vi "print HP.vi"(0 "peaks graph 1":cluster{cluster{"X":dbl, "Y":dbl}[]}[](graph)=[{[{"X"=0.0, "Y"=88.0}, {"X"=0.05, "Y"=88.0}, {"X"=0.1, "Y"=87.0}, {"X"=0.15000000000000002, "Y"=87.0}, {"X"=0.2, "Y"=88.0}, {"X"=0.25, "Y"=88.0}, {"X"=0.30000000000000004, "Y"=88.0}, {"X"=0.35000000000000003, "Y"=87.0}, {"X"=0.4, "Y"=88.0}, {"X"=0.45, "Y"=87.0}, {"X"=0.5, "Y"=88.0}, {"X"=0.55, "Y"=88.0}, {"X"=0.6000000000000001, "Y"=88.0}, {"X"=0.65, "Y"=88.0}, {"X"=0.7000000000000001, "Y"=87.0}, {"X"=0.75, "Y"=88.0}, {"X"=0.8, "Y"=88.0}, {"X"=0.8500000000000001, "Y"=88.0}, {"X"=0.9, "Y"=87.0}, {"X"=0.9500000000000001, "Y"=88.0}, {"X"=1.0, "Y"=88.0}, {"X"=1.05, "Y"=88.0}, {"X"=1.1, "Y"=87.0}, {"X"=1.1500000000000001, "Y"=87.0}, {"X"=1.2000000000000002, "Y"=87.0}, {"X"=1.25, "Y"=88.0}, {"X"=1.3, "Y"=88.0}, {"X"=1.35, "Y"=87.0}, {"X"=1.4000000000000001, "Y"=87.0}, {"X"=1.4500000000000002, "Y"=88.0}, {"X"=1.5, "Y"=87.0}, {"X"=1.55, "Y"=88.0}, {"X"=1.6, "Y"=88.0}, {"X"=1.6500000000000001, "Y"=87.0}, {"X"=1.7000000000000002, "Y"=87.0}, {"X"=1.75, "Y"=87.0}, {"X"=1.8, "Y"=88.0}, {"X"=1.85, "Y"=88.0}, {"X"=1.9000000000000001, "Y"=88.0}, {"X"=1.9500000000000002, "Y"=87.0}, {"X"=2.0, "Y"=88.0}, {"X"=2.0500000000000003, "Y"=87.0}, {"X"=2.1, "Y"=87.0}, {"X"=2.15, "Y"=88.0}, {"X"=2.2, "Y"=88.0}, {"X"=2.25, "Y"=87.0}, {"X"=2.3000000000000003, "Y"=88.0}, {"X"=2.35, "Y"=88.0}, {"X"=2.4000000000000004, "Y"=88.0}, {"X"=2.45, "Y"=87.0}, {"X"=2.5, "Y"=88.0}, {"X"=2.5500000000000003, "Y"=88.0}, {"X"=2.6, "Y"=87.0}, {"X"=2.6500000000000004, "Y"=87.0}, {"X"=2.7, "Y"=87.0}, {"X"=2.75, "Y"=87.0}, {"X"=2.8000000000000003, "Y"=87.0}, {"X"=2.85, "Y"=87.0}, {"X"=2.9000000000000004, "Y"=87.0}, {"X"=2.95, "Y"=87.0}, {"X"=3.0, "Y"=87.0}, {"X"=3.0500000000000003, "Y"=87.0}, {"X"=3.1, "Y"=87.0}, {"X"=3.1500000000000004, "Y"=88.0}, {"X"=3.2, "Y"=87.0}, {"X"=3.25, "Y"=88.0}, {"X"=3.3000000000000003, "Y"=87.0}, {"X"=3.35, "Y"=87.0}, {"X"=3.4000000000000004, "Y"=87.0}, {"X"=3.45, "Y"=87.0}, {"X"=3.5, "Y"=88.0}, {"X"=3.5500000000000003, "Y"=87.0}, {"X"=3.6, "Y"=87.0}, {"X"=3.6500000000000004, "Y"=87.0}, {"X"=3.7, "Y"=88.0}, {"X"=3.75, "Y"=87.0}, {"X"=3.8000000000000003, "Y"=88.0}, {"X"=3.85, "Y"=87.0}, {"X"=3.9000000000000004, "Y"=87.0}, {"X"=3.95, "Y"=88.0}, {"X"=4.0, "Y"=88.0}, {"X"=4.05, "Y"=88.0}, {"X"=4.1000000000000005, "Y"=88.0}, {"X"=4.15, "Y"=88.0}, {"X"=4.2, "Y"=88.0}, {"X"=4.25, "Y"=87.0}, {"X"=4.3, "Y"=87.0}, {"X"=4.3500000000000005, "Y"=88.0}, {"X"=4.4, "Y"=87.0}, {"X"=4.45, "Y"=87.0}, {"X"=4.5, "Y"=88.0}, {"X"=4.55, "Y"=87.0}, {"X"=4.6000000000000005, "Y"=87.0}, {"X"=4.65, "Y"=87.0}, {"X"=4.7, "Y"=87.0}, {"X"=4.75, "Y"=88.0}, {"X"=4.800000000000001, "Y"=88.0}, {"X"=4.8500000000000005, "Y"=88.0}, {"X"=4.9, "Y"=87.0}, {"X"=4.95, "Y"=87.0}, {"X"=5.0, "Y"=88.0}, {"X"=5.050000000000001, "Y"=88.0}, {"X"=5.1000000000000005, "Y"=88.0}, {"X"=5.15, "Y"=87.0}, {"X"=5.2, "Y"=88.0}, {"X"=5.25, "Y"=88.0}, {"X"=5.300000000000001, "Y"=88.0}, {"X"=5.3500000000000005, "Y"=87.0}, {"X"=5.4, "Y"=87.0}, {"X"=5.45, "Y"=87.0}, {"X"=5.5, "Y"=88.0}, {"X"=5.550000000000001, "Y"=87.0}, {"X"=5.6000000000000005, "Y"=88.0}, {"X"=5.65, "Y"=88.0}, {"X"=5.7, "Y"=88.0}, {"X"=5.75, "Y"=87.0}, {"X"=5.800000000000001, "Y"=89.0}, {"X"=5.8500000000000005, "Y"=87.0}, {"X"=5.9, "Y"=88.0}, {"X"=5.95, "Y"=88.0}, {"X"=6.0, "Y"=88.0}, {"X"=6.050000000000001, "Y"=88.0}, {"X"=6.1000000000000005, "Y"=88.0}, {"X"=6.15, "Y"=87.0}, {"X"=6.2, "Y"=88.0}, {"X"=6.25, "Y"=88.0}, {"X"=6.300000000000001, "Y"=87.0}, {"X"=6.3500000000000005, "Y"=87.0}, {"X"=6.4, "Y"=88.0}, {"X"=6.45, "Y"=87.0}, {"X"=6.5, "Y"=88.0}, {"X"=6.550000000000001, "Y"=87.0}, {"X"=6.6000000000000005, "Y"=87.0}, {"X"=6.65, "Y"=88.0}, {"X"=6.7, "Y"=87.0}, {"X"=6.75, "Y"=88.0}, {"X"=6.800000000000001, "Y"=88.0}, {"X"=6.8500000000000005, "Y"=88.0}, {"X"=6.9, "Y"=87.0}, {"X"=6.95, "Y"=87.0}, {"X"=7.0, "Y"=87.0}, {"X"=7.050000000000001, "Y"=87.0}, {"X"=7.1000000000000005, "Y"=87.0}, {"X"=7.15, "Y"=87.0}, {"X"=7.2, "Y"=87.0}, {"X"=7.25, "Y"=88.0}, {"X"=7.300000000000001, "Y"=87.0}, {"X"=7.3500000000000005, "Y"=87.0}, {"X"=7.4, "Y"=88.0}, {"X"=7.45, "Y"=87.0}, {"X"=7.5, "Y"=88.0}, {"X"=7.550000000000001, "Y"=88.0}, {"X"=7.6000000000000005, "Y"=87.0}, {"X"=7.65, "Y"=87.0}, {"X"=7.7, "Y"=87.0}, {"X"=7.75, "Y"=87.0}, {"X"=7.800000000000001, "Y"=87.0}, {"X"=7.8500000000000005, "Y"=87.0}, {"X"=7.9, "Y"=87.0}, {"X"=7.95, "Y"=88.0}, {"X"=8.0, "Y"=88.0}, {"X"=8.05, "Y"=87.0}, {"X"=8.1, "Y"=88.0}, {"X"=8.15, "Y"=87.0}, {"X"=8.200000000000001, "Y"=87.0}, {"X"=8.25, "Y"=87.0}, {"X"=8.3, "Y"=87.0}, {"X"=8.35, "Y"=86.0}, {"X"=8.4, "Y"=87.0}, {"X"=8.450000000000001, "Y"=87.0}, {"X"=8.5, "Y"=87.0}, {"X"=8.55, "Y"=87.0}, {"X"=8.6, "Y"=86.0}, {"X"=8.65, "Y"=87.0}, {"X"=8.700000000000001, "Y"=86.0}, {"X"=8.75, "Y"=87.0}, {"X"=8.8, "Y"=87.0}, {"X"=8.85, "Y"=87.0}, {"X"=8.9, "Y"=86.0}, {"X"=8.950000000000001, "Y"=86.0}, {"X"=9.0, "Y"=87.0}, {"X"=9.05, "Y"=87.0}, {"X"=9.1, "Y"=88.0}, {"X"=9.15, "Y"=87.0}, {"X"=9.200000000000001, "Y"=87.0}, {"X"=9.25, "Y"=87.0}, {"X"=9.3, "Y"=87.0}, {"X"=9.35, "Y"=87.0}, {"X"=9.4, "Y"=88.0}, {"X"=9.450000000000001, "Y"=87.0}, {"X"=9.5, "Y"=88.0}, {"X"=9.55, "Y"=87.0}, {"X"=9.600000000000001, "Y"=87.0}, {"X"=9.65, "Y"=87.0}, {"X"=9.700000000000001, "Y"=87.0}, {"X"=9.75, "Y"=87.0}, {"X"=9.8, "Y"=87.0}, {"X"=9.850000000000001, "Y"=87.0}, {"X"=9.9, "Y"=87.0}, {"X"=9.950000000000001, "Y"=87.0}, {"X"=10.0, "Y"=87.0}, {"X"=10.05, "Y"=88.0}, {"X"=10.100000000000001, "Y"=88.0}, {"X"=10.15, "Y"=88.0}, {"X"=10.200000000000001, "Y"=87.0}, {"X"=10.25, "Y"=87.0}, {"X"=10.3, "Y"=88.0}, {"X"=10.350000000000001, "Y"=88.0}, {"X"=10.4, "Y"=88.0}, {"X"=10.450000000000001, "Y"=87.0}, {"X"=10.5, "Y"=88.0}, {"X"=10.55, "Y"=88.0}, {"X"=10.600000000000001, "Y"=88.0}, {"X"=10.65, "Y"=87.0}, {"X"=10.700000000000001, "Y"=88.0}, {"X"=10.75, "Y"=88.0}, {"X"=10.8, "Y"=88.0}, {"X"=10.850000000000001, "Y"=87.0}, {"X"=10.9, "Y"=88.0}, {"X"=10.950000000000001, "Y"=88.0}, {"X"=11.0, "Y"=88.0}, {"X"=11.05, "Y"=88.0}, {"X"=11.100000000000001, "Y"=88.0}, {"X"=11.15, "Y"=88.0}, {"X"=11.200000000000001, "Y"=87.0}, {"X"=11.25, "Y"=87.0}, {"X"=11.3, "Y"=88.0}, {"X"=11.350000000000001, "Y"=87.0}, {"X"=11.4, "Y"=87.0}, {"X"=11.450000000000001, "Y"=87.0}, {"X"=11.5, "Y"=87.0}, {"X"=11.55, "Y"=87.0}, {"X"=11.600000000000001, "Y"=87.0}, {"X"=11.65, "Y"=87.0}, {"X"=11.700000000000001, "Y"=87.0}, {"X"=11.75, "Y"=87.0}, {"X"=11.8, "Y"=87.0}, {"X"=11.850000000000001, "Y"=86.0}, {"X"=11.9, "Y"=87.0}, {"X"=11.950000000000001, "Y"=87.0}, {"X"=12.0, "Y"=87.0}, {"X"=12.05, "Y"=87.0}, {"X"=12.100000000000001, "Y"=87.0}, {"X"=12.15, "Y"=87.0}, {"X"=12.200000000000001, "Y"=87.0}, {"X"=12.25, "Y"=87.0}, {"X"=12.3, "Y"=87.0}, {"X"=12.350000000000001, "Y"=87.0}, {"X"=12.4, "Y"=87.0}, {"X"=12.450000000000001, "Y"=87.0}, {"X"=12.5, "Y"=87.0}, {"X"=12.55, "Y"=87.0}, {"X"=12.600000000000001, "Y"=88.0}, {"X"=12.65, "Y"=87.0}, {"X"=12.700000000000001, "Y"=87.0}, {"X"=12.75, "Y"=87.0}, {"X"=12.8, "Y"=88.0}, {"X"=12.850000000000001, "Y"=87.0}, {"X"=12.9, "Y"=87.0}, {"X"=12.950000000000001, "Y"=87.0}, {"X"=13.0, "Y"=88.0}, {"X"=13.05, "Y"=87.0}, {"X"=13.100000000000001, "Y"=88.0}, {"X"=13.15, "Y"=88.0}, {"X"=13.200000000000001, "Y"=87.0}, {"X"=13.25, "Y"=87.0}, {"X"=13.3, "Y"=87.0}, {"X"=13.350000000000001, "Y"=88.0}, {"X"=13.4, "Y"=87.0}, {"X"=13.450000000000001, "Y"=87.0}, {"X"=13.5, "Y"=87.0}, {"X"=13.55, "Y"=87.0}, {"X"=13.600000000000001, "Y"=87.0}, {"X"=13.65, "Y"=87.0}, {"X"=13.700000000000001, "Y"=87.0}, {"X"=13.75, "Y"=87.0}, {"X"=13.8, "Y"=88.0}, {"X"=13.850000000000001, "Y"=87.0}, {"X"=13.9, "Y"=87.0}, {"X"=13.950000000000001, "Y"=87.0}, {"X"=14.0, "Y"=88.0}, {"X"=14.05, "Y"=88.0}, {"X"=14.100000000000001, "Y"=87.0}, {"X"=14.15, "Y"=87.0}, {"X"=14.200000000000001, "Y"=87.0}, {"X"=14.25, "Y"=87.0}, {"X"=14.3, "Y"=88.0}, {"X"=14.350000000000001, "Y"=87.0}, {"X"=14.4, "Y"=87.0}, {"X"=14.450000000000001, "Y"=87.0}, {"X"=14.5, "Y"=87.0}, {"X"=14.55, "Y"=87.0}, {"X"=14.600000000000001, "Y"=87.0}, {"X"=14.65, "Y"=87.0}, {"X"=14.700000000000001, "Y"=87.0}, {"X"=14.75, "Y"=87.0}, {"X"=14.8, "Y"=86.0}, {"X"=14.850000000000001, "Y"=86.0}, {"X"=14.9, "Y"=87.0}, {"X"=14.950000000000001, "Y"=87.0}, {"X"=15.0, "Y"=87.0}, {"X"=15.05, "Y"=86.0}, {"X"=15.100000000000001, "Y"=87.0}, {"X"=15.15, "Y"=87.0}, {"X"=15.200000000000001, "Y"=87.0}, {"X"=15.25, "Y"=87.0}, {"X"=15.3, "Y"=87.0}, {"X"=15.350000000000001, "Y"=87.0}, {"X"=15.4, "Y"=87.0}, {"X"=15.450000000000001, "Y"=87.0}, {"X"=15.5, "Y"=88.0}, {"X"=15.55, "Y"=87.0}, {"X"=15.600000000000001, "Y"=88.0}, {"X"=15.65, "Y"=87.0}, {"X"=15.700000000000001, "Y"=88.0}, {"X"=15.75, "Y"=88.0}, {"X"=15.8, "Y"=87.0}, {"X"=15.850000000000001, "Y"=88.0}, {"X"=15.9, "Y"=88.0}, {"X"=15.950000000000001, "Y"=88.0}, {"X"=16.0, "Y"=87.0}, {"X"=16.05, "Y"=88.0}, {"X"=16.1, "Y"=88.0}, {"X"=16.150000000000002, "Y"=87.0}, {"X"=16.2, "Y"=87.0}, {"X"=16.25, "Y"=87.0}, {"X"=16.3, "Y"=87.0}, {"X"=16.35, "Y"=88.0}, {"X"=16.400000000000002, "Y"=87.0}, {"X"=16.45, "Y"=87.0}, {"X"=16.5, "Y"=88.0}, {"X"=16.55, "Y"=88.0}, {"X"=16.6, "Y"=86.0}, {"X"=16.650000000000002, "Y"=85.0}, {"X"=16.7, "Y"=84.0}, {"X"=16.75, "Y"=84.0}, {"X"=16.8, "Y"=84.0}, {"X"=16.85, "Y"=84.0}, {"X"=16.900000000000002, "Y"=84.0}, {"X"=16.95, "Y"=84.0}, {"X"=17.0, "Y"=85.0}, {"X"=17.05, "Y"=85.0}, {"X"=17.1, "Y"=85.0}, {"X"=17.150000000000002, "Y"=85.0}, {"X"=17.2, "Y"=86.0}, {"X"=17.25, "Y"=85.0}, {"X"=17.3, "Y"=86.0}, {"X"=17.35, "Y"=85.0}, {"X"=17.400000000000002, "Y"=86.0}, {"X"=17.45, "Y"=85.0}, {"X"=17.5, "Y"=86.0}, {"X"=17.55, "Y"=86.0}, {"X"=17.6, "Y"=87.0}, {"X"=17.650000000000002, "Y"=87.0}, {"X"=17.7, "Y"=87.0}, {"X"=17.75, "Y"=88.0}, {"X"=17.8, "Y"=87.0}, {"X"=17.85, "Y"=88.0}, {"X"=17.900000000000002, "Y"=89.0}, {"X"=17.95, "Y"=89.0}, {"X"=18.0, "Y"=90.0}, {"X"=18.05, "Y"=90.0}, {"X"=18.1, "Y"=91.0}, {"X"=18.150000000000002, "Y"=91.0}, {"X"=18.2, "Y"=91.0}, {"X"=18.25, "Y"=92.0}, {"X"=18.3, "Y"=93.0}, {"X"=18.35, "Y"=92.0}, {"X"=18.400000000000002, "Y"=92.0}, {"X"=18.45, "Y"=93.0}, {"X"=18.5, "Y"=93.0}, {"X"=18.55, "Y"=93.0}, {"X"=18.6, "Y"=93.0}, {"X"=18.650000000000002, "Y"=93.0}, {"X"=18.7, "Y"=95.0}, {"X"=18.75, "Y"=94.0}, {"X"=18.8, "Y"=95.0}, {"X"=18.85, "Y"=94.0}, {"X"=18.900000000000002, "Y"=97.0}, {"X"=18.95, "Y"=134.0}, {"X"=19.0, "Y"=1494.0}, {"X"=19.05, "Y"=9292.0}, {"X"=19.1, "Y"=22149.0}, {"X"=19.150000000000002, "Y"=25427.0}, {"X"=19.200000000000003, "Y"=16419.0}, {"X"=19.25, "Y"=8793.0}, {"X"=19.3, "Y"=6892.0}, {"X"=19.35, "Y"=6644.0}, {"X"=19.400000000000002, "Y"=7200.0}, {"X"=19.450000000000003, "Y"=11546.0}, {"X"=19.5, "Y"=21745.0}, {"X"=19.55, "Y"=32369.0}, {"X"=19.6, "Y"=37093.0}, {"X"=19.650000000000002, "Y"=37317.0}, {"X"=19.700000000000003, "Y"=36691.0}, {"X"=19.75, "Y"=36232.0}, {"X"=19.8, "Y"=35896.0}, {"X"=19.85, "Y"=35616.0}, {"X"=19.900000000000002, "Y"=35359.0}, {"X"=19.950000000000003, "Y"=35089.0}, {"X"=20.0, "Y"=34786.0}, {"X"=20.05, "Y"=34454.0}, {"X"=20.1, "Y"=34100.0}, {"X"=20.150000000000002, "Y"=33726.0}, {"X"=20.200000000000003, "Y"=33337.0}, {"X"=20.25, "Y"=32952.0}, {"X"=20.3, "Y"=32584.0}, {"X"=20.35, "Y"=32244.0}, {"X"=20.400000000000002, "Y"=31934.0}, {"X"=20.450000000000003, "Y"=31635.0}, {"X"=20.5, "Y"=31332.0}, {"X"=20.55, "Y"=31043.0}, {"X"=20.6, "Y"=30811.0}, {"X"=20.650000000000002, "Y"=30627.0}, {"X"=20.700000000000003, "Y"=30451.0}, {"X"=20.75, "Y"=30266.0}, {"X"=20.8, "Y"=30077.0}, {"X"=20.85, "Y"=29881.0}, {"X"=20.900000000000002, "Y"=29695.0}, {"X"=20.950000000000003, "Y"=29529.0}, {"X"=21.0, "Y"=29328.0}, {"X"=21.05, "Y"=29053.0}, {"X"=21.1, "Y"=28830.0}, {"X"=21.150000000000002, "Y"=28774.0}, {"X"=21.200000000000003, "Y"=28761.0}, {"X"=21.25, "Y"=28650.0}, {"X"=21.3, "Y"=28499.0}, {"X"=21.35, "Y"=28330.0}, {"X"=21.400000000000002, "Y"=28073.0}, {"X"=21.450000000000003, "Y"=27738.0}, {"X"=21.5, "Y"=27362.0}, {"X"=21.55, "Y"=27064.0}, {"X"=21.6, "Y"=27024.0}, {"X"=21.650000000000002, "Y"=27151.0}, {"X"=21.700000000000003, "Y"=27170.0}, {"X"=21.75, "Y"=27027.0}, {"X"=21.8, "Y"=26824.0}, {"X"=21.85, "Y"=26577.0}, {"X"=21.900000000000002, "Y"=26071.0}, {"X"=21.950000000000003, "Y"=24628.0}, {"X"=22.0, "Y"=21372.0}, {"X"=22.05, "Y"=15864.0}, {"X"=22.1, "Y"=9100.0}, {"X"=22.150000000000002, "Y"=3744.0}, {"X"=22.200000000000003, "Y"=1373.0}, {"X"=22.25, "Y"=887.0}, {"X"=22.3, "Y"=840.0}, {"X"=22.35, "Y"=823.0}, {"X"=22.400000000000002, "Y"=811.0}, {"X"=22.450000000000003, "Y"=802.0}, {"X"=22.5, "Y"=789.0}, {"X"=22.55, "Y"=773.0}, {"X"=22.6, "Y"=756.0}, {"X"=22.650000000000002, "Y"=737.0}, {"X"=22.700000000000003, "Y"=717.0}, {"X"=22.75, "Y"=695.0}, {"X"=22.8, "Y"=675.0}, {"X"=22.85, "Y"=655.0}, {"X"=22.900000000000002, "Y"=636.0}, {"X"=22.950000000000003, "Y"=617.0}, {"X"=23.0, "Y"=599.0}, {"X"=23.05, "Y"=579.0}, {"X"=23.1, "Y"=561.0}, {"X"=23.150000000000002, "Y"=543.0}, {"X"=23.200000000000003, "Y"=526.0}, {"X"=23.25, "Y"=510.0}, {"X"=23.3, "Y"=495.0}, {"X"=23.35, "Y"=480.0}, {"X"=23.400000000000002, "Y"=465.0}, {"X"=23.450000000000003, "Y"=452.0}, {"X"=23.5, "Y"=437.0}, {"X"=23.55, "Y"=424.0}, {"X"=23.6, "Y"=411.0}, {"X"=23.650000000000002, "Y"=400.0}, {"X"=23.700000000000003, "Y"=387.0}, {"X"=23.75, "Y"=374.0}, {"X"=23.8, "Y"=363.0}, {"X"=23.85, "Y"=352.0}, {"X"=23.900000000000002, "Y"=342.0}, {"X"=23.950000000000003, "Y"=331.0}, {"X"=24.0, "Y"=322.0}, {"X"=24.05, "Y"=311.0}, {"X"=24.1, "Y"=302.0}, {"X"=24.150000000000002, "Y"=293.0}, {"X"=24.200000000000003, "Y"=285.0}, {"X"=24.25, "Y"=276.0}, {"X"=24.3, "Y"=268.0}, {"X"=24.35, "Y"=260.0}, {"X"=24.400000000000002, "Y"=253.0}, {"X"=24.450000000000003, "Y"=246.0}, {"X"=24.5, "Y"=239.0}, {"X"=24.55, "Y"=232.0}, {"X"=24.6, "Y"=226.0}, {"X"=24.650000000000002, "Y"=219.0}, {"X"=24.700000000000003, "Y"=213.0}, {"X"=24.75, "Y"=207.0}, {"X"=24.8, "Y"=203.0}, {"X"=24.85, "Y"=197.0}, {"X"=24.900000000000002, "Y"=193.0}, {"X"=24.950000000000003, "Y"=188.0}, {"X"=25.0, "Y"=190.0}, {"X"=25.05, "Y"=370.0}, {"X"=25.1, "Y"=2421.0}, {"X"=25.150000000000002, "Y"=7244.0}, {"X"=25.200000000000003, "Y"=10319.0}, {"X"=25.25, "Y"=8486.0}, {"X"=25.3, "Y"=5587.0}, {"X"=25.35, "Y"=4463.0}, {"X"=25.400000000000002, "Y"=4232.0}, {"X"=25.450000000000003, "Y"=4409.0}, {"X"=25.5, "Y"=5909.0}, {"X"=25.55, "Y"=9591.0}, {"X"=25.6, "Y"=13714.0}, {"X"=25.650000000000002, "Y"=15772.0}, {"X"=25.700000000000003, "Y"=16034.0}, {"X"=25.75, "Y"=15898.0}, {"X"=25.8, "Y"=15813.0}, {"X"=25.85, "Y"=15770.0}, {"X"=25.900000000000002, "Y"=15743.0}, {"X"=25.950000000000003, "Y"=15721.0}, {"X"=26.0, "Y"=15700.0}, {"X"=26.05, "Y"=15677.0}, {"X"=26.1, "Y"=15660.0}, {"X"=26.150000000000002, "Y"=15647.0}, {"X"=26.200000000000003, "Y"=15634.0}, {"X"=26.25, "Y"=15617.0}, {"X"=26.3, "Y"=15598.0}, {"X"=26.35, "Y"=15577.0}, {"X"=26.400000000000002, "Y"=15559.0}, {"X"=26.450000000000003, "Y"=15540.0}, {"X"=26.5, "Y"=15522.0}, {"X"=26.55, "Y"=15504.0}, {"X"=26.6, "Y"=15485.0}, {"X"=26.650000000000002, "Y"=15461.0}, {"X"=26.700000000000003, "Y"=15440.0}, {"X"=26.75, "Y"=15427.0}, {"X"=26.8, "Y"=15410.0}, {"X"=26.85, "Y"=15384.0}, {"X"=26.900000000000002, "Y"=15358.0}, {"X"=26.950000000000003, "Y"=15335.0}, {"X"=27.0, "Y"=15314.0}, {"X"=27.05, "Y"=15292.0}, {"X"=27.1, "Y"=15271.0}, {"X"=27.150000000000002, "Y"=15248.0}, {"X"=27.200000000000003, "Y"=15226.0}, {"X"=27.25, "Y"=15206.0}, {"X"=27.3, "Y"=15184.0}, {"X"=27.35, "Y"=15157.0}, {"X"=27.400000000000002, "Y"=15133.0}, {"X"=27.450000000000003, "Y"=15107.0}, {"X"=27.5, "Y"=15084.0}, {"X"=27.55, "Y"=15076.0}, {"X"=27.6, "Y"=272511.0}, {"X"=27.650000000000002, "Y"=12734285.0}, {"X"=27.700000000000003, "Y"=52991102.0}, {"X"=27.75, "Y"=86340386.0}, {"X"=27.8, "Y"=64463573.0}, {"X"=27.85, "Y"=19785049.0}, {"X"=27.900000000000002, "Y"=1140097.0}, {"X"=27.950000000000003, "Y"=49.0}, {"X"=28.0, "Y"=44.0}, {"X"=28.05, "Y"=43.0}, {"X"=28.1, "Y"=46.0}, {"X"=28.150000000000002, "Y"=84.0}, {"X"=28.200000000000003, "Y"=239.0}, {"X"=28.25, "Y"=528.0}, {"X"=28.3, "Y"=812.0}, {"X"=28.35, "Y"=947.0}, {"X"=28.400000000000002, "Y"=957.0}, {"X"=28.450000000000003, "Y"=918.0}, {"X"=28.5, "Y"=867.0}, {"X"=28.55, "Y"=815.0}, {"X"=28.6, "Y"=765.0}, {"X"=28.650000000000002, "Y"=721.0}, {"X"=28.700000000000003, "Y"=680.0}, {"X"=28.75, "Y"=642.0}, {"X"=28.8, "Y"=609.0}, {"X"=28.85, "Y"=577.0}, {"X"=28.900000000000002, "Y"=547.0}, {"X"=28.950000000000003, "Y"=520.0}, {"X"=29.0, "Y"=495.0}, {"X"=29.05, "Y"=474.0}, {"X"=29.1, "Y"=452.0}, {"X"=29.150000000000002, "Y"=432.0}, {"X"=29.200000000000003, "Y"=414.0}, {"X"=29.25, "Y"=396.0}, {"X"=29.3, "Y"=379.0}, {"X"=29.35, "Y"=363.0}, {"X"=29.400000000000002, "Y"=346.0}, {"X"=29.450000000000003, "Y"=332.0}, {"X"=29.5, "Y"=318.0}, {"X"=29.55, "Y"=305.0}, {"X"=29.6, "Y"=292.0}, {"X"=29.650000000000002, "Y"=281.0}, {"X"=29.700000000000003, "Y"=270.0}, {"X"=29.75, "Y"=260.0}, {"X"=29.8, "Y"=251.0}, {"X"=29.85, "Y"=241.0}, {"X"=29.900000000000002, "Y"=232.0}, {"X"=29.950000000000003, "Y"=222.0}, {"X"=30.0, "Y"=215.0}, {"X"=30.05, "Y"=208.0}, {"X"=30.1, "Y"=200.0}, {"X"=30.150000000000002, "Y"=193.0}, {"X"=30.200000000000003, "Y"=186.0}, {"X"=30.25, "Y"=179.0}, {"X"=30.3, "Y"=172.0}, {"X"=30.35, "Y"=167.0}, {"X"=30.400000000000002, "Y"=161.0}, {"X"=30.450000000000003, "Y"=157.0}, {"X"=30.5, "Y"=151.0}, {"X"=30.55, "Y"=145.0}, {"X"=30.6, "Y"=139.0}, {"X"=30.650000000000002, "Y"=135.0}, {"X"=30.700000000000003, "Y"=132.0}, {"X"=30.75, "Y"=128.0}, {"X"=30.8, "Y"=123.0}, {"X"=30.85, "Y"=119.0}, {"X"=30.900000000000002, "Y"=115.0}, {"X"=30.950000000000003, "Y"=111.0}, {"X"=31.0, "Y"=108.0}, {"X"=31.05, "Y"=105.0}, {"X"=31.1, "Y"=102.0}, {"X"=31.150000000000002, "Y"=97.0}, {"X"=31.200000000000003, "Y"=95.0}, {"X"=31.25, "Y"=94.0}, {"X"=31.3, "Y"=91.0}, {"X"=31.35, "Y"=86.0}, {"X"=31.400000000000002, "Y"=85.0}, {"X"=31.450000000000003, "Y"=83.0}, {"X"=31.5, "Y"=80.0}, {"X"=31.55, "Y"=76.0}, {"X"=31.6, "Y"=74.0}, {"X"=31.650000000000002, "Y"=73.0}, {"X"=31.700000000000003, "Y"=72.0}, {"X"=31.75, "Y"=69.0}, {"X"=31.8, "Y"=66.0}, {"X"=31.85, "Y"=64.0}, {"X"=31.900000000000002, "Y"=63.0}, {"X"=31.950000000000003, "Y"=63.0}, {"X"=32.0, "Y"=62.0}, {"X"=32.050000000000004, "Y"=59.0}, {"X"=32.1, "Y"=57.0}, {"X"=32.15, "Y"=54.0}, {"X"=32.2, "Y"=54.0}, {"X"=32.25, "Y"=54.0}, {"X"=32.300000000000004, "Y"=53.0}, {"X"=32.35, "Y"=53.0}, {"X"=32.4, "Y"=50.0}, {"X"=32.45, "Y"=46.0}, {"X"=32.5, "Y"=46.0}, {"X"=32.550000000000004, "Y"=45.0}, {"X"=32.6, "Y"=45.0}, {"X"=32.65, "Y"=45.0}, {"X"=32.7, "Y"=45.0}, {"X"=32.75, "Y"=43.0}, {"X"=32.800000000000004, "Y"=42.0}, {"X"=32.85, "Y"=39.0}, {"X"=32.9, "Y"=37.0}, {"X"=32.95, "Y"=38.0}, {"X"=33.0, "Y"=37.0}, {"X"=33.050000000000004, "Y"=38.0}, {"X"=33.1, "Y"=37.0}, {"X"=33.15, "Y"=37.0}, {"X"=33.2, "Y"=37.0}, {"X"=33.25, "Y"=34.0}, {"X"=33.300000000000004, "Y"=32.0}, {"X"=33.35, "Y"=31.0}, {"X"=33.4, "Y"=30.0}, {"X"=33.45, "Y"=30.0}, {"X"=33.5, "Y"=30.0}, {"X"=33.550000000000004, "Y"=30.0}, {"X"=33.6, "Y"=30.0}, {"X"=33.65, "Y"=30.0}, {"X"=33.7, "Y"=29.0}, {"X"=33.75, "Y"=29.0}, {"X"=33.800000000000004, "Y"=25.0}, {"X"=33.85, "Y"=25.0}, {"X"=33.9, "Y"=24.0}, {"X"=33.95, "Y"=24.0}, {"X"=34.0, "Y"=24.0}, {"X"=34.050000000000004, "Y"=24.0}, {"X"=34.1, "Y"=24.0}, {"X"=34.15, "Y"=24.0}, {"X"=34.2, "Y"=23.0}, {"X"=34.25, "Y"=24.0}, {"X"=34.300000000000004, "Y"=22.0}, {"X"=34.35, "Y"=21.0}, {"X"=34.4, "Y"=19.0}, {"X"=34.45, "Y"=18.0}, {"X"=34.5, "Y"=18.0}, {"X"=34.550000000000004, "Y"=18.0}, {"X"=34.6, "Y"=18.0}, {"X"=34.65, "Y"=18.0}, {"X"=34.7, "Y"=18.0}, {"X"=34.75, "Y"=18.0}, {"X"=34.800000000000004, "Y"=18.0}, {"X"=34.85, "Y"=16.0}, {"X"=34.9, "Y"=16.0}, {"X"=34.95, "Y"=14.0}, {"X"=35.0, "Y"=13.0}, {"X"=35.050000000000004, "Y"=14.0}, {"X"=35.1, "Y"=13.0}, {"X"=35.15, "Y"=14.0}, {"X"=35.2, "Y"=13.0}, {"X"=35.25, "Y"=13.0}, {"X"=35.300000000000004, "Y"=13.0}, {"X"=35.35, "Y"=12.0}, {"X"=35.4, "Y"=11.0}, {"X"=35.45, "Y"=10.0}, {"X"=35.5, "Y"=9.0}, {"X"=35.550000000000004, "Y"=9.0}, {"X"=35.6, "Y"=9.0}, {"X"=35.65, "Y"=9.0}, {"X"=35.7, "Y"=9.0}, {"X"=35.75, "Y"=9.0}, {"X"=35.800000000000004, "Y"=9.0}, {"X"=35.85, "Y"=9.0}, {"X"=35.9, "Y"=9.0}, {"X"=35.95, "Y"=9.0}, {"X"=36.0, "Y"=9.0}, {"X"=36.050000000000004, "Y"=9.0}, {"X"=36.1, "Y"=8.0}, {"X"=36.15, "Y"=8.0}, {"X"=36.2, "Y"=8.0}, {"X"=36.25, "Y"=7.0}, {"X"=36.300000000000004, "Y"=8.0}, {"X"=36.35, "Y"=7.0}, {"X"=36.4, "Y"=8.0}, {"X"=36.45, "Y"=7.0}, {"X"=36.5, "Y"=8.0}, {"X"=36.550000000000004, "Y"=7.0}, {"X"=36.6, "Y"=7.0}, {"X"=36.65, "Y"=7.0}, {"X"=36.7, "Y"=7.0}, {"X"=36.75, "Y"=6.0}, {"X"=36.800000000000004, "Y"=7.0}, {"X"=36.85, "Y"=7.0}, {"X"=36.9, "Y"=7.0}, {"X"=36.95, "Y"=6.0}, {"X"=37.0, "Y"=7.0}, {"X"=37.050000000000004, "Y"=7.0}, {"X"=37.1, "Y"=6.0}, {"X"=37.15, "Y"=6.0}, {"X"=37.2, "Y"=7.0}, {"X"=37.25, "Y"=6.0}, {"X"=37.300000000000004, "Y"=6.0}, {"X"=37.35, "Y"=6.0}, {"X"=37.4, "Y"=6.0}, {"X"=37.45, "Y"=6.0}, {"X"=37.5, "Y"=6.0}, {"X"=37.550000000000004, "Y"=6.0}, {"X"=37.6, "Y"=6.0}, {"X"=37.65, "Y"=6.0}, {"X"=37.7, "Y"=6.0}, {"X"=37.75, "Y"=6.0}, {"X"=37.800000000000004, "Y"=6.0}, {"X"=37.85, "Y"=6.0}, {"X"=37.9, "Y"=6.0}, {"X"=37.95, "Y"=6.0}, {"X"=38.0, "Y"=5.0}, {"X"=38.050000000000004, "Y"=6.0}, {"X"=38.1, "Y"=5.0}, {"X"=38.15, "Y"=5.0}, {"X"=38.2, "Y"=471187.0}, {"X"=38.25, "Y"=3859300.0}, {"X"=38.300000000000004, "Y"=10408589.0}, {"X"=38.35, "Y"=13956745.0}, {"X"=38.400000000000006, "Y"=12087206.0}, {"X"=38.45, "Y"=9724769.0}, {"X"=38.5, "Y"=9023885.0}, {"X"=38.550000000000004, "Y"=8780700.0}, {"X"=38.6, "Y"=8557695.0}, {"X"=38.650000000000006, "Y"=8382895.0}, {"X"=38.7, "Y"=8404163.0}, {"X"=38.75, "Y"=12247328.0}, {"X"=38.800000000000004, "Y"=28939746.0}, {"X"=38.85, "Y"=57648728.0}, {"X"=38.900000000000006, "Y"=80110212.0}, {"X"=38.95, "Y"=86206370.0}, {"X"=39.0, "Y"=83953263.0}, {"X"=39.050000000000004, "Y"=80679646.0}, {"X"=39.1, "Y"=77489411.0}, {"X"=39.150000000000006, "Y"=74393162.0}, {"X"=39.2, "Y"=71389721.0}, {"X"=39.25, "Y"=68476477.0}, {"X"=39.300000000000004, "Y"=65650861.0}, {"X"=39.35, "Y"=62910482.0}, {"X"=39.400000000000006, "Y"=60253744.0}, {"X"=39.45, "Y"=57680377.0}, {"X"=39.5, "Y"=55190464.0}, {"X"=39.550000000000004, "Y"=52781972.0}, {"X"=39.6, "Y"=50451825.0}, {"X"=39.650000000000006, "Y"=48199887.0}, {"X"=39.7, "Y"=46027264.0}, {"X"=39.75, "Y"=43931992.0}, {"X"=39.800000000000004, "Y"=41911356.0}, {"X"=39.85, "Y"=39965512.0}, {"X"=39.900000000000006, "Y"=38095214.0}, {"X"=39.95, "Y"=36298049.0}, {"X"=40.0, "Y"=34570187.0}, {"X"=40.050000000000004, "Y"=32912273.0}, {"X"=40.1, "Y"=31328723.0}, {"X"=40.150000000000006, "Y"=29818510.0}, {"X"=40.2, "Y"=28374298.0}, {"X"=40.25, "Y"=26993368.0}, {"X"=40.300000000000004, "Y"=25677890.0}, {"X"=40.35, "Y"=24425119.0}, {"X"=40.400000000000006, "Y"=23230064.0}, {"X"=40.45, "Y"=22092028.0}, {"X"=40.5, "Y"=21011263.0}, {"X"=40.550000000000004, "Y"=19986014.0}, {"X"=40.6, "Y"=19013278.0}, {"X"=40.650000000000006, "Y"=18090074.0}, {"X"=40.7, "Y"=17215653.0}, {"X"=40.75, "Y"=16389852.0}, {"X"=40.800000000000004, "Y"=15609582.0}, {"X"=40.85, "Y"=14870994.0}, {"X"=40.900000000000006, "Y"=14172000.0}, {"X"=40.95, "Y"=13511075.0}, {"X"=41.0, "Y"=12886722.0}, {"X"=41.050000000000004, "Y"=12297686.0}, {"X"=41.1, "Y"=11742847.0}, {"X"=41.150000000000006, "Y"=11220172.0}, {"X"=41.2, "Y"=10726463.0}, {"X"=41.25, "Y"=10259724.0}, {"X"=41.300000000000004, "Y"=9819587.0}, {"X"=41.35, "Y"=9405046.0}, {"X"=41.400000000000006, "Y"=9014227.0}, {"X"=41.45, "Y"=8645638.0}, {"X"=41.5, "Y"=8298142.0}, {"X"=41.550000000000004, "Y"=7970622.0}, {"X"=41.6, "Y"=7662471.0}, {"X"=41.650000000000006, "Y"=7373623.0}, {"X"=41.7, "Y"=7103387.0}, {"X"=41.75, "Y"=6849742.0}, {"X"=41.800000000000004, "Y"=6610547.0}, {"X"=41.85, "Y"=6385028.0}, {"X"=41.900000000000006, "Y"=6173224.0}, {"X"=41.95, "Y"=5974400.0}, {"X"=42.0, "Y"=5787094.0}, {"X"=42.050000000000004, "Y"=5610652.0}, {"X"=42.1, "Y"=5445212.0}, {"X"=42.150000000000006, "Y"=5290469.0}, {"X"=42.2, "Y"=5145522.0}, {"X"=42.25, "Y"=5009316.0}, {"X"=42.300000000000004, "Y"=4881111.0}, {"X"=42.35, "Y"=4760412.0}, {"X"=42.400000000000006, "Y"=4646468.0}, {"X"=42.45, "Y"=4538548.0}, {"X"=42.5, "Y"=4436403.0}, {"X"=42.550000000000004, "Y"=4340269.0}, {"X"=42.6, "Y"=4250640.0}, {"X"=42.650000000000006, "Y"=4167326.0}, {"X"=42.7, "Y"=4088805.0}, {"X"=42.75, "Y"=4013782.0}, {"X"=42.800000000000004, "Y"=3942599.0}, {"X"=42.85, "Y"=3876084.0}, {"X"=42.900000000000006, "Y"=3814028.0}, {"X"=42.95, "Y"=3755575.0}, {"X"=43.0, "Y"=3700346.0}, {"X"=43.050000000000004, "Y"=3648410.0}, {"X"=43.1, "Y"=3599567.0}, {"X"=43.150000000000006, "Y"=3553074.0}, {"X"=43.2, "Y"=3508238.0}, {"X"=43.25, "Y"=3465350.0}, {"X"=43.300000000000004, "Y"=3425341.0}, {"X"=43.35, "Y"=3388464.0}, {"X"=43.400000000000006, "Y"=3353881.0}, {"X"=43.45, "Y"=3320622.0}, {"X"=43.5, "Y"=3288709.0}, {"X"=43.550000000000004, "Y"=3258557.0}, {"X"=43.6, "Y"=3229890.0}, {"X"=43.650000000000006, "Y"=3202230.0}, {"X"=43.7, "Y"=3175720.0}, {"X"=43.75, "Y"=3150589.0}, {"X"=43.800000000000004, "Y"=3126174.0}, {"X"=43.85, "Y"=3101636.0}, {"X"=43.900000000000006, "Y"=3077496.0}, {"X"=43.95, "Y"=3054926.0}, {"X"=44.0, "Y"=3034039.0}, {"X"=44.050000000000004, "Y"=3014177.0}, {"X"=44.1, "Y"=2994989.0}, {"X"=44.150000000000006, "Y"=2976505.0}, {"X"=44.2, "Y"=2958527.0}, {"X"=44.25, "Y"=2940729.0}, {"X"=44.300000000000004, "Y"=2923239.0}, {"X"=44.35, "Y"=2906377.0}, {"X"=44.400000000000006, "Y"=2890251.0}, {"X"=44.45, "Y"=2874752.0}, {"X"=44.5, "Y"=2859474.0}, {"X"=44.550000000000004, "Y"=2844225.0}, {"X"=44.6, "Y"=2829471.0}, {"X"=44.650000000000006, "Y"=2815546.0}, {"X"=44.7, "Y"=2802103.0}, {"X"=44.75, "Y"=2788660.0}, {"X"=44.800000000000004, "Y"=2775052.0}, {"X"=44.85, "Y"=2761452.0}, {"X"=44.900000000000006, "Y"=2748068.0}, {"X"=44.95, "Y"=2734866.0}, {"X"=45.0, "Y"=2721862.0}, {"X"=45.050000000000004, "Y"=2709332.0}, {"X"=45.1, "Y"=2697425.0}, {"X"=45.150000000000006, "Y"=2685974.0}, {"X"=45.2, "Y"=2674698.0}, {"X"=45.25, "Y"=2663394.0}, {"X"=45.300000000000004, "Y"=2652066.0}, {"X"=45.35, "Y"=2640847.0}, {"X"=45.400000000000006, "Y"=2629693.0}, {"X"=45.45, "Y"=2618451.0}, {"X"=45.5, "Y"=2607472.0}, {"X"=45.550000000000004, "Y"=2597298.0}, {"X"=45.6, "Y"=2587729.0}, {"X"=45.650000000000006, "Y"=2578141.0}, {"X"=45.7, "Y"=2568319.0}, {"X"=45.75, "Y"=2558377.0}, {"X"=45.800000000000004, "Y"=2548390.0}, {"X"=45.85, "Y"=2538485.0}, {"X"=45.900000000000006, "Y"=2528991.0}, {"X"=45.95, "Y"=2519978.0}, {"X"=46.0, "Y"=2511196.0}, {"X"=46.050000000000004, "Y"=2502540.0}, {"X"=46.1, "Y"=2493771.0}, {"X"=46.150000000000006, "Y"=2484451.0}, {"X"=46.2, "Y"=2474695.0}, {"X"=46.25, "Y"=2465294.0}, {"X"=46.300000000000004, "Y"=2456705.0}, {"X"=46.35, "Y"=2448706.0}, {"X"=46.400000000000006, "Y"=2440887.0}, {"X"=46.45, "Y"=2432757.0}, {"X"=46.5, "Y"=2424294.0}, {"X"=46.550000000000004, "Y"=2415966.0}, {"X"=46.6, "Y"=2407734.0}, {"X"=46.650000000000006, "Y"=2399413.0}, {"X"=46.7, "Y"=2391163.0}, {"X"=46.75, "Y"=2382933.0}, {"X"=46.800000000000004, "Y"=2374532.0}, {"X"=46.85, "Y"=2366039.0}, {"X"=46.900000000000006, "Y"=2357583.0}, {"X"=46.95, "Y"=2349067.0}, {"X"=47.0, "Y"=2340667.0}, {"X"=47.050000000000004, "Y"=2332895.0}, {"X"=47.1, "Y"=2325605.0}, {"X"=47.150000000000006, "Y"=2318144.0}, {"X"=47.2, "Y"=2310443.0}, {"X"=47.25, "Y"=2302706.0}, {"X"=47.300000000000004, "Y"=2294808.0}, {"X"=47.35, "Y"=2286614.0}, {"X"=47.400000000000006, "Y"=2278256.0}, {"X"=47.45, "Y"=2270013.0}, {"X"=47.5, "Y"=2261937.0}, {"X"=47.550000000000004, "Y"=2253798.0}, {"X"=47.6, "Y"=2245705.0}, {"X"=47.650000000000006, "Y"=2237950.0}, {"X"=47.7, "Y"=2230438.0}, {"X"=47.75, "Y"=2222987.0}, {"X"=47.800000000000004, "Y"=2215495.0}, {"X"=47.85, "Y"=2208050.0}, {"X"=47.900000000000006, "Y"=2200779.0}, {"X"=47.95, "Y"=2193391.0}, {"X"=48.0, "Y"=2185953.0}, {"X"=48.050000000000004, "Y"=2179011.0}, {"X"=48.1, "Y"=2172318.0}, {"X"=48.150000000000006, "Y"=2165271.0}, {"X"=48.2, "Y"=2158066.0}, {"X"=48.25, "Y"=2151080.0}, {"X"=48.300000000000004, "Y"=2144157.0}, {"X"=48.35, "Y"=2137044.0}, {"X"=48.400000000000006, "Y"=2129859.0}, {"X"=48.45, "Y"=2122948.0}, {"X"=48.5, "Y"=2116317.0}, {"X"=48.550000000000004, "Y"=2109555.0}, {"X"=48.6, "Y"=2102570.0}, {"X"=48.650000000000006, "Y"=2095765.0}, {"X"=48.7, "Y"=2089208.0}, {"X"=48.75, "Y"=2082491.0}, {"X"=48.800000000000004, "Y"=2075512.0}, {"X"=48.85, "Y"=2068614.0}, {"X"=48.900000000000006, "Y"=2062020.0}, {"X"=48.95, "Y"=2055600.0}, {"X"=49.0, "Y"=2049148.0}, {"X"=49.050000000000004, "Y"=2042722.0}, {"X"=49.1, "Y"=2036522.0}, {"X"=49.150000000000006, "Y"=2030381.0}, {"X"=49.2, "Y"=2024026.0}, {"X"=49.25, "Y"=2017758.0}, {"X"=49.300000000000004, "Y"=2011863.0}, {"X"=49.35, "Y"=2005945.0}, {"X"=49.400000000000006, "Y"=1999927.0}, {"X"=49.45, "Y"=1994273.0}, {"X"=49.5, "Y"=1988859.0}, {"X"=49.550000000000004, "Y"=1983325.0}, {"X"=49.6, "Y"=1977838.0}, {"X"=49.650000000000006, "Y"=1972500.0}, {"X"=49.7, "Y"=1967140.0}, {"X"=49.75, "Y"=1961695.0}, {"X"=49.800000000000004, "Y"=1956204.0}, {"X"=49.85, "Y"=1950683.0}, {"X"=49.900000000000006, "Y"=1945123.0}, {"X"=49.95, "Y"=1939565.0}, {"X"=50.0, "Y"=1934023.0}, {"X"=50.050000000000004, "Y"=1928430.0}, {"X"=50.1, "Y"=1922901.0}, {"X"=50.150000000000006, "Y"=1917590.0}, {"X"=50.2, "Y"=1912349.0}, {"X"=50.25, "Y"=1907006.0}, {"X"=50.300000000000004, "Y"=1901705.0}, {"X"=50.35, "Y"=1896644.0}, {"X"=50.400000000000006, "Y"=1891622.0}, {"X"=50.45, "Y"=1886253.0}, {"X"=50.5, "Y"=1880676.0}, {"X"=50.550000000000004, "Y"=1875380.0}, {"X"=50.6, "Y"=1870506.0}, {"X"=50.650000000000006, "Y"=1865871.0}, {"X"=50.7, "Y"=1861322.0}, {"X"=50.75, "Y"=1856756.0}, {"X"=50.800000000000004, "Y"=1852102.0}, {"X"=50.85, "Y"=1847333.0}, {"X"=50.900000000000006, "Y"=1842459.0}, {"X"=50.95, "Y"=1837569.0}, {"X"=51.0, "Y"=1832751.0}, {"X"=51.050000000000004, "Y"=1828007.0}, {"X"=51.1, "Y"=1823374.0}, {"X"=51.150000000000006, "Y"=1818756.0}, {"X"=51.2, "Y"=1813729.0}, {"X"=51.25, "Y"=1808151.0}, {"X"=51.300000000000004, "Y"=1802616.0}, {"X"=51.35, "Y"=1797680.0}, {"X"=51.400000000000006, "Y"=1793068.0}, {"X"=51.45, "Y"=1788310.0}, {"X"=51.5, "Y"=1783511.0}, {"X"=51.550000000000004, "Y"=1778872.0}, {"X"=51.6, "Y"=1774111.0}, {"X"=51.650000000000006, "Y"=1768961.0}, {"X"=51.7, "Y"=1763720.0}, {"X"=51.75, "Y"=1758697.0}, {"X"=51.800000000000004, "Y"=1753886.0}, {"X"=51.85, "Y"=1749332.0}, {"X"=51.900000000000006, "Y"=1745068.0}, {"X"=51.95, "Y"=1741005.0}, {"X"=52.0, "Y"=1736896.0}, {"X"=52.050000000000004, "Y"=1732583.0}, {"X"=52.1, "Y"=1728220.0}, {"X"=52.150000000000006, "Y"=1723771.0}, {"X"=52.2, "Y"=1718995.0}, {"X"=52.25, "Y"=1713918.0}, {"X"=52.300000000000004, "Y"=1708671.0}, {"X"=52.35, "Y"=1703383.0}, {"X"=52.400000000000006, "Y"=1698285.0}, {"X"=52.45, "Y"=1693567.0}, {"X"=52.5, "Y"=1689229.0}, {"X"=52.550000000000004, "Y"=1685143.0}, {"X"=52.6, "Y"=1681025.0}, {"X"=52.650000000000006, "Y"=1676621.0}, {"X"=52.7, "Y"=1671981.0}, {"X"=52.75, "Y"=1667299.0}, {"X"=52.800000000000004, "Y"=1662792.0}, {"X"=52.85, "Y"=1658638.0}, {"X"=52.900000000000006, "Y"=1654742.0}, {"X"=52.95, "Y"=1650854.0}, {"X"=53.0, "Y"=1646915.0}, {"X"=53.050000000000004, "Y"=1642999.0}, {"X"=53.1, "Y"=1639107.0}, {"X"=53.150000000000006, "Y"=1635119.0}, {"X"=53.2, "Y"=1630915.0}, {"X"=53.25, "Y"=1626510.0}, {"X"=53.300000000000004, "Y"=1621891.0}, {"X"=53.35, "Y"=1617185.0}, {"X"=53.400000000000006, "Y"=1612852.0}, {"X"=53.45, "Y"=1609031.0}, {"X"=53.5, "Y"=1605259.0}, {"X"=53.550000000000004, "Y"=1601118.0}, {"X"=53.6, "Y"=1596679.0}, {"X"=53.650000000000006, "Y"=1592195.0}, {"X"=53.7, "Y"=1587664.0}, {"X"=53.75, "Y"=1583072.0}, {"X"=53.800000000000004, "Y"=1578630.0}, {"X"=53.85, "Y"=1574274.0}, {"X"=53.900000000000006, "Y"=1569598.0}, {"X"=53.95, "Y"=1564675.0}, {"X"=54.0, "Y"=1560130.0}, {"X"=54.050000000000004, "Y"=1556063.0}, {"X"=54.1, "Y"=1551911.0}, {"X"=54.150000000000006, "Y"=1547456.0}, {"X"=54.2, "Y"=1543082.0}, {"X"=54.25, "Y"=1538979.0}, {"X"=54.300000000000004, "Y"=1534740.0}, {"X"=54.35, "Y"=1530156.0}, {"X"=54.400000000000006, "Y"=1525587.0}, {"X"=54.45, "Y"=1521059.0}, {"X"=54.5, "Y"=1516366.0}, {"X"=54.550000000000004, "Y"=1511736.0}, {"X"=54.6, "Y"=1507375.0}, {"X"=54.650000000000006, "Y"=1503100.0}, {"X"=54.7, "Y"=1498693.0}, {"X"=54.75, "Y"=1494241.0}, {"X"=54.800000000000004, "Y"=1489940.0}, {"X"=54.85, "Y"=1485633.0}, {"X"=54.900000000000006, "Y"=1481072.0}, {"X"=54.95, "Y"=1476407.0}, {"X"=55.0, "Y"=1471850.0}, {"X"=55.050000000000004, "Y"=1467293.0}, {"X"=55.1, "Y"=1462551.0}, {"X"=55.150000000000006, "Y"=1457704.0}, {"X"=55.2, "Y"=1453091.0}, {"X"=55.25, "Y"=1448874.0}, {"X"=55.300000000000004, "Y"=1444924.0}, {"X"=55.35, "Y"=1440983.0}, {"X"=55.400000000000006, "Y"=1436866.0}, {"X"=55.45, "Y"=1432576.0}, {"X"=55.5, "Y"=1428127.0}, {"X"=55.550000000000004, "Y"=1423580.0}, {"X"=55.6, "Y"=1419068.0}, {"X"=55.650000000000006, "Y"=1414502.0}, {"X"=55.7, "Y"=1409769.0}, {"X"=55.75, "Y"=1405120.0}, {"X"=55.800000000000004, "Y"=1400790.0}, {"X"=55.85, "Y"=1396554.0}, {"X"=55.900000000000006, "Y"=1392243.0}, {"X"=55.95, "Y"=1388087.0}, {"X"=56.0, "Y"=1384118.0}, {"X"=56.050000000000004, "Y"=1379977.0}, {"X"=56.1, "Y"=1375500.0}, {"X"=56.150000000000006, "Y"=1371002.0}, {"X"=56.2, "Y"=1366769.0}, {"X"=56.25, "Y"=1362672.0}, {"X"=56.300000000000004, "Y"=1358546.0}, {"X"=56.35, "Y"=1354450.0}, {"X"=56.400000000000006, "Y"=1350424.0}, {"X"=56.45, "Y"=1346302.0}, {"X"=56.5, "Y"=1341939.0}, {"X"=56.550000000000004, "Y"=1337331.0}, {"X"=56.6, "Y"=1332463.0}, {"X"=56.650000000000006, "Y"=1327549.0}, {"X"=56.7, "Y"=1322841.0}, {"X"=56.75, "Y"=1318268.0}, {"X"=56.800000000000004, "Y"=1313727.0}, {"X"=56.85, "Y"=1309247.0}, {"X"=56.900000000000006, "Y"=1304892.0}, {"X"=56.95, "Y"=1300628.0}, {"X"=57.0, "Y"=1296340.0}, {"X"=57.050000000000004, "Y"=1292031.0}, {"X"=57.1, "Y"=1287720.0}, {"X"=57.150000000000006, "Y"=1283346.0}, {"X"=57.2, "Y"=1278932.0}, {"X"=57.25, "Y"=1274548.0}, {"X"=57.300000000000004, "Y"=1270259.0}, {"X"=57.35, "Y"=1266144.0}, {"X"=57.400000000000006, "Y"=1262182.0}, {"X"=57.45, "Y"=1258221.0}, {"X"=57.5, "Y"=1254190.0}, {"X"=57.550000000000004, "Y"=1250056.0}, {"X"=57.6, "Y"=1245746.0}, {"X"=57.650000000000006, "Y"=1241397.0}, {"X"=57.7, "Y"=1237163.0}, {"X"=57.75, "Y"=1232917.0}, {"X"=57.800000000000004, "Y"=1228586.0}, {"X"=57.85, "Y"=1224346.0}, {"X"=57.900000000000006, "Y"=1220247.0}, {"X"=57.95, "Y"=1216077.0}, {"X"=58.0, "Y"=1211865.0}, {"X"=58.050000000000004, "Y"=1207907.0}, {"X"=58.1, "Y"=1204149.0}, {"X"=58.150000000000006, "Y"=1200241.0}, {"X"=58.2, "Y"=1196271.0}, {"X"=58.25, "Y"=1192510.0}, {"X"=58.300000000000004, "Y"=1188776.0}, {"X"=58.35, "Y"=1184884.0}, {"X"=58.400000000000006, "Y"=1180979.0}, {"X"=58.45, "Y"=1177270.0}, {"X"=58.5, "Y"=1173771.0}, {"X"=58.550000000000004, "Y"=1170183.0}, {"X"=58.6, "Y"=1166373.0}, {"X"=58.650000000000006, "Y"=1162607.0}, {"X"=58.7, "Y"=1158989.0}, {"X"=58.75, "Y"=1155366.0}, {"X"=58.800000000000004, "Y"=1151656.0}, {"X"=58.85, "Y"=1147898.0}, {"X"=58.900000000000006, "Y"=1144136.0}, {"X"=58.95, "Y"=1140360.0}, {"X"=59.0, "Y"=1136668.0}, {"X"=59.050000000000004, "Y"=1133185.0}, {"X"=59.1, "Y"=1129819.0}, {"X"=59.150000000000006, "Y"=1126403.0}, {"X"=59.2, "Y"=1122919.0}, {"X"=59.25, "Y"=1119525.0}, {"X"=59.300000000000004, "Y"=1116271.0}, {"X"=59.35, "Y"=1113023.0}, {"X"=59.400000000000006, "Y"=1109726.0}, {"X"=59.45, "Y"=1106445.0}, {"X"=59.5, "Y"=1103213.0}, {"X"=59.550000000000004, "Y"=1099994.0}, {"X"=59.6, "Y"=1096723.0}, {"X"=59.650000000000006, "Y"=1093412.0}, {"X"=59.7, "Y"=1090150.0}, {"X"=59.75, "Y"=1086961.0}, {"X"=59.800000000000004, "Y"=1083848.0}, {"X"=59.85, "Y"=1080773.0}, {"X"=59.900000000000006, "Y"=1077551.0}, {"X"=59.95, "Y"=1074183.0}, {"X"=60.0, "Y"=1070912.0}, {"X"=60.050000000000004, "Y"=1067779.0}, {"X"=60.1, "Y"=1064690.0}, {"X"=60.150000000000006, "Y"=1061659.0}, {"X"=60.2, "Y"=1058711.0}, {"X"=60.25, "Y"=1055927.0}, {"X"=60.300000000000004, "Y"=1053277.0}, {"X"=60.35, "Y"=1050459.0}, {"X"=60.400000000000006, "Y"=1047435.0}, {"X"=60.45, "Y"=1044541.0}, {"X"=60.5, "Y"=1041886.0}, {"X"=60.550000000000004, "Y"=1039316.0}, {"X"=60.6, "Y"=1036627.0}, {"X"=60.650000000000006, "Y"=1033750.0}, {"X"=60.7, "Y"=1030950.0}, {"X"=60.75, "Y"=1028434.0}, {"X"=60.800000000000004, "Y"=1025978.0}, {"X"=60.85, "Y"=1023293.0}, {"X"=60.900000000000006, "Y"=1020363.0}, {"X"=60.95, "Y"=1017366.0}, {"X"=61.0, "Y"=1014503.0}, {"X"=61.050000000000004, "Y"=1011822.0}, {"X"=61.1, "Y"=1009173.0}, {"X"=61.150000000000006, "Y"=1006374.0}, {"X"=61.2, "Y"=1003492.0}, {"X"=61.25, "Y"=1000745.0}, {"X"=61.300000000000004, "Y"=998153.0}, {"X"=61.35, "Y"=995635.0}, {"X"=61.400000000000006, "Y"=993147.0}, {"X"=61.45, "Y"=990629.0}, {"X"=61.5, "Y"=988096.0}, {"X"=61.550000000000004, "Y"=985642.0}, {"X"=61.6, "Y"=983267.0}, {"X"=61.650000000000006, "Y"=980875.0}, {"X"=61.7, "Y"=978431.0}, {"X"=61.75, "Y"=975986.0}, {"X"=61.800000000000004, "Y"=973594.0}, {"X"=61.85, "Y"=971248.0}, {"X"=61.900000000000006, "Y"=968882.0}, {"X"=61.95, "Y"=966447.0}, {"X"=62.0, "Y"=963939.0}, {"X"=62.050000000000004, "Y"=961427.0}, {"X"=62.1, "Y"=959029.0}, {"X"=62.150000000000006, "Y"=956720.0}, {"X"=62.2, "Y"=954385.0}, {"X"=62.25, "Y"=952004.0}, {"X"=62.300000000000004, "Y"=949645.0}, {"X"=62.35, "Y"=947340.0}, {"X"=62.400000000000006, "Y"=945086.0}, {"X"=62.45, "Y"=942849.0}, {"X"=62.5, "Y"=940533.0}, {"X"=62.550000000000004, "Y"=938134.0}, {"X"=62.6, "Y"=935785.0}, {"X"=62.650000000000006, "Y"=933548.0}, {"X"=62.7, "Y"=931396.0}, {"X"=62.75, "Y"=929290.0}, {"X"=62.800000000000004, "Y"=927250.0}, {"X"=62.85, "Y"=925324.0}, {"X"=62.900000000000006, "Y"=923425.0}, {"X"=62.95, "Y"=921368.0}, {"X"=63.0, "Y"=919153.0}, {"X"=63.050000000000004, "Y"=916930.0}, {"X"=63.1, "Y"=914788.0}, {"X"=63.150000000000006, "Y"=912718.0}, {"X"=63.2, "Y"=910691.0}, {"X"=63.25, "Y"=908706.0}, {"X"=63.300000000000004, "Y"=906742.0}, {"X"=63.35, "Y"=904742.0}, {"X"=63.400000000000006, "Y"=902694.0}, {"X"=63.45, "Y"=900638.0}, {"X"=63.5, "Y"=898623.0}, {"X"=63.550000000000004, "Y"=896559.0}, {"X"=63.6, "Y"=894379.0}, {"X"=63.650000000000006, "Y"=892162.0}, {"X"=63.7, "Y"=889926.0}, {"X"=63.75, "Y"=887752.0}, {"X"=63.800000000000004, "Y"=885776.0}, {"X"=63.85, "Y"=883897.0}, {"X"=63.900000000000006, "Y"=881863.0}, {"X"=63.95, "Y"=879692.0}, {"X"=64.0, "Y"=877600.0}, {"X"=64.05, "Y"=875662.0}, {"X"=64.10000000000001, "Y"=873816.0}, {"X"=64.15, "Y"=871979.0}, {"X"=64.2, "Y"=870050.0}, {"X"=64.25, "Y"=868037.0}, {"X"=64.3, "Y"=866007.0}, {"X"=64.35000000000001, "Y"=863980.0}, {"X"=64.4, "Y"=861973.0}, {"X"=64.45, "Y"=860031.0}, {"X"=64.5, "Y"=858113.0}, {"X"=64.55, "Y"=856081.0}, {"X"=64.60000000000001, "Y"=853967.0}, {"X"=64.65, "Y"=851956.0}, {"X"=64.7, "Y"=850048.0}, {"X"=64.75, "Y"=848144.0}, {"X"=64.8, "Y"=846220.0}, {"X"=64.85000000000001, "Y"=844308.0}, {"X"=64.9, "Y"=842458.0}, {"X"=64.95, "Y"=840632.0}, {"X"=65.0, "Y"=838737.0}, {"X"=65.05, "Y"=836810.0}, {"X"=65.10000000000001, "Y"=834966.0}, {"X"=65.15, "Y"=833226.0}, {"X"=65.2, "Y"=831525.0}, {"X"=65.25, "Y"=829817.0}, {"X"=65.3, "Y"=828088.0}, {"X"=65.35000000000001, "Y"=826338.0}, {"X"=65.4, "Y"=824575.0}, {"X"=65.45, "Y"=822828.0}, {"X"=65.5, "Y"=821100.0}, {"X"=65.55, "Y"=819355.0}, {"X"=65.60000000000001, "Y"=817547.0}, {"X"=65.65, "Y"=815649.0}, {"X"=65.7, "Y"=813694.0}, {"X"=65.75, "Y"=811760.0}, {"X"=65.8, "Y"=809949.0}, {"X"=65.85000000000001, "Y"=808334.0}, {"X"=65.9, "Y"=806831.0}, {"X"=65.95, "Y"=805288.0}, {"X"=66.0, "Y"=803662.0}, {"X"=66.05, "Y"=801948.0}, {"X"=66.10000000000001, "Y"=800130.0}, {"X"=66.15, "Y"=798251.0}, {"X"=66.2, "Y"=796442.0}, {"X"=66.25, "Y"=794842.0}, {"X"=66.3, "Y"=793395.0}, {"X"=66.35000000000001, "Y"=791936.0}, {"X"=66.4, "Y"=790455.0}, {"X"=66.45, "Y"=788966.0}, {"X"=66.5, "Y"=787367.0}, {"X"=66.55, "Y"=785617.0}, {"X"=66.60000000000001, "Y"=783823.0}, {"X"=66.65, "Y"=782145.0}, {"X"=66.7, "Y"=780598.0}, {"X"=66.75, "Y"=779027.0}, {"X"=66.8, "Y"=777382.0}, {"X"=66.85000000000001, "Y"=775725.0}, {"X"=66.9, "Y"=774017.0}, {"X"=66.95, "Y"=772248.0}, {"X"=67.0, "Y"=770586.0}, {"X"=67.05, "Y"=769142.0}, {"X"=67.10000000000001, "Y"=767833.0}, {"X"=67.15, "Y"=766518.0}, {"X"=67.2, "Y"=765114.0}, {"X"=67.25, "Y"=763671.0}, {"X"=67.3, "Y"=762239.0}, {"X"=67.35000000000001, "Y"=760722.0}, {"X"=67.4, "Y"=759093.0}, {"X"=67.45, "Y"=757539.0}, {"X"=67.5, "Y"=756198.0}, {"X"=67.55, "Y"=754845.0}, {"X"=67.60000000000001, "Y"=753274.0}, {"X"=67.65, "Y"=751679.0}, {"X"=67.7, "Y"=750184.0}, {"X"=67.75, "Y"=748696.0}, {"X"=67.8, "Y"=747192.0}, {"X"=67.85000000000001, "Y"=745682.0}, {"X"=67.9, "Y"=744223.0}, {"X"=67.95, "Y"=742827.0}, {"X"=68.0, "Y"=741300.0}, {"X"=68.05, "Y"=739579.0}, {"X"=68.10000000000001, "Y"=737831.0}, {"X"=68.15, "Y"=736142.0}, {"X"=68.2, "Y"=734513.0}, {"X"=68.25, "Y"=733016.0}, {"X"=68.3, "Y"=731660.0}, {"X"=68.35000000000001, "Y"=730316.0}, {"X"=68.4, "Y"=728937.0}, {"X"=68.45, "Y"=727565.0}, {"X"=68.5, "Y"=726162.0}, {"X"=68.55, "Y"=724667.0}, {"X"=68.60000000000001, "Y"=723157.0}, {"X"=68.65, "Y"=721803.0}, {"X"=68.7, "Y"=720644.0}, {"X"=68.75, "Y"=719541.0}, {"X"=68.8, "Y"=718326.0}, {"X"=68.85000000000001, "Y"=716956.0}, {"X"=68.9, "Y"=715521.0}, {"X"=68.95, "Y"=714084.0}, {"X"=69.0, "Y"=712656.0}, {"X"=69.05, "Y"=711318.0}, {"X"=69.10000000000001, "Y"=710051.0}, {"X"=69.15, "Y"=708726.0}, {"X"=69.2, "Y"=707317.0}, {"X"=69.25, "Y"=705927.0}, {"X"=69.3, "Y"=704631.0}, {"X"=69.35000000000001, "Y"=703380.0}, {"X"=69.4, "Y"=702085.0}, {"X"=69.45, "Y"=700783.0}, {"X"=69.5, "Y"=699581.0}, {"X"=69.55, "Y"=698557.0}, {"X"=69.60000000000001, "Y"=697631.0}, {"X"=69.65, "Y"=696623.0}, {"X"=69.7, "Y"=695536.0}, {"X"=69.75, "Y"=694482.0}, {"X"=69.8, "Y"=693452.0}, {"X"=69.85000000000001, "Y"=692349.0}, {"X"=69.9, "Y"=691185.0}, {"X"=69.95, "Y"=690049.0}, {"X"=70.0, "Y"=688968.0}, {"X"=70.05, "Y"=687916.0}, {"X"=70.10000000000001, "Y"=686830.0}, {"X"=70.15, "Y"=685653.0}, {"X"=70.2, "Y"=684397.0}, {"X"=70.25, "Y"=683072.0}, {"X"=70.3, "Y"=681635.0}, {"X"=70.35000000000001, "Y"=680091.0}, {"X"=70.4, "Y"=678613.0}, {"X"=70.45, "Y"=677383.0}, {"X"=70.5, "Y"=676370.0}, {"X"=70.55, "Y"=675397.0}, {"X"=70.60000000000001, "Y"=674365.0}, {"X"=70.65, "Y"=673337.0}, {"X"=70.7, "Y"=672337.0}, {"X"=70.75, "Y"=671291.0}, {"X"=70.8, "Y"=670166.0}, {"X"=70.85000000000001, "Y"=668960.0}, {"X"=70.9, "Y"=667727.0}, {"X"=70.95, "Y"=666583.0}, {"X"=71.0, "Y"=665516.0}, {"X"=71.05, "Y"=664393.0}, {"X"=71.10000000000001, "Y"=663178.0}, {"X"=71.15, "Y"=661996.0}, {"X"=71.2, "Y"=660991.0}, {"X"=71.25, "Y"=660141.0}, {"X"=71.3, "Y"=659264.0}, {"X"=71.35000000000001, "Y"=658253.0}, {"X"=71.4, "Y"=657176.0}, {"X"=71.45, "Y"=656105.0}, {"X"=71.5, "Y"=655005.0}, {"X"=71.55, "Y"=653815.0}, {"X"=71.60000000000001, "Y"=652533.0}, {"X"=71.65, "Y"=651263.0}, {"X"=71.7, "Y"=650102.0}, {"X"=71.75, "Y"=649056.0}, {"X"=71.8, "Y"=648079.0}, {"X"=71.85000000000001, "Y"=647138.0}, {"X"=71.9, "Y"=646227.0}, {"X"=71.95, "Y"=645302.0}, {"X"=72.0, "Y"=644343.0}, {"X"=72.05, "Y"=643393.0}, {"X"=72.10000000000001, "Y"=642444.0}, {"X"=72.15, "Y"=641438.0}, {"X"=72.2, "Y"=640335.0}, {"X"=72.25, "Y"=639198.0}, {"X"=72.3, "Y"=638179.0}, {"X"=72.35000000000001, "Y"=637313.0}, {"X"=72.4, "Y"=636470.0}, {"X"=72.45, "Y"=635542.0}, {"X"=72.5, "Y"=634494.0}, {"X"=72.55, "Y"=633310.0}, {"X"=72.60000000000001, "Y"=632081.0}, {"X"=72.65, "Y"=630968.0}, {"X"=72.7, "Y"=630007.0}, {"X"=72.75, "Y"=629074.0}, {"X"=72.8, "Y"=628092.0}, {"X"=72.85000000000001, "Y"=627157.0}, {"X"=72.9, "Y"=626335.0}, {"X"=72.95, "Y"=625514.0}, {"X"=73.0, "Y"=624540.0}, {"X"=73.05, "Y"=623420.0}, {"X"=73.10000000000001, "Y"=622346.0}, {"X"=73.15, "Y"=621374.0}, {"X"=73.2, "Y"=620362.0}, {"X"=73.25, "Y"=619324.0}, {"X"=73.3, "Y"=618429.0}, {"X"=73.35000000000001, "Y"=617608.0}, {"X"=73.4, "Y"=616631.0}, {"X"=73.45, "Y"=615563.0}, {"X"=73.5, "Y"=614607.0}, {"X"=73.55, "Y"=613751.0}, {"X"=73.60000000000001, "Y"=612877.0}, {"X"=73.65, "Y"=611901.0}, {"X"=73.7, "Y"=610812.0}, {"X"=73.75, "Y"=609729.0}, {"X"=73.8, "Y"=608734.0}, {"X"=73.85000000000001, "Y"=607799.0}, {"X"=73.9, "Y"=606836.0}, {"X"=73.95, "Y"=605800.0}, {"X"=74.0, "Y"=604739.0}, {"X"=74.05, "Y"=603743.0}, {"X"=74.10000000000001, "Y"=602860.0}, {"X"=74.15, "Y"=602071.0}, {"X"=74.2, "Y"=601320.0}, {"X"=74.25, "Y"=600550.0}, {"X"=74.3, "Y"=599762.0}, {"X"=74.35000000000001, "Y"=598971.0}, {"X"=74.4, "Y"=598149.0}, {"X"=74.45, "Y"=597248.0}, {"X"=74.5, "Y"=596291.0}, {"X"=74.55, "Y"=595340.0}, {"X"=74.60000000000001, "Y"=594416.0}, {"X"=74.65, "Y"=593517.0}, {"X"=74.7, "Y"=592622.0}, {"X"=74.75, "Y"=591694.0}, {"X"=74.8, "Y"=590676.0}, {"X"=74.85000000000001, "Y"=589597.0}, {"X"=74.9, "Y"=588601.0}, {"X"=74.95, "Y"=587708.0}, {"X"=75.0, "Y"=586849.0}, {"X"=75.05, "Y"=586074.0}, {"X"=75.10000000000001, "Y"=585354.0}, {"X"=75.15, "Y"=584559.0}, {"X"=75.2, "Y"=583693.0}, {"X"=75.25, "Y"=582799.0}, {"X"=75.3, "Y"=581937.0}, {"X"=75.35000000000001, "Y"=581132.0}, {"X"=75.4, "Y"=580309.0}, {"X"=75.45, "Y"=579434.0}, {"X"=75.5, "Y"=578567.0}, {"X"=75.55, "Y"=577709.0}, {"X"=75.60000000000001, "Y"=576774.0}, {"X"=75.65, "Y"=575778.0}, {"X"=75.7, "Y"=574832.0}, {"X"=75.75, "Y"=573959.0}, {"X"=75.8, "Y"=573091.0}, {"X"=75.85000000000001, "Y"=572160.0}, {"X"=75.9, "Y"=571203.0}, {"X"=75.95, "Y"=570285.0}, {"X"=76.0, "Y"=569361.0}, {"X"=76.05, "Y"=568408.0}, {"X"=76.10000000000001, "Y"=567489.0}, {"X"=76.15, "Y"=566643.0}, {"X"=76.2, "Y"=565800.0}, {"X"=76.25, "Y"=564877.0}, {"X"=76.3, "Y"=563926.0}, {"X"=76.35000000000001, "Y"=563063.0}, {"X"=76.4, "Y"=562261.0}, {"X"=76.45, "Y"=561432.0}, {"X"=76.5, "Y"=560575.0}, {"X"=76.55, "Y"=559746.0}, {"X"=76.60000000000001, "Y"=558905.0}, {"X"=76.65, "Y"=557926.0}, {"X"=76.7, "Y"=556845.0}, {"X"=76.75, "Y"=555839.0}, {"X"=76.80000000000001, "Y"=554956.0}, {"X"=76.85000000000001, "Y"=554092.0}, {"X"=76.9, "Y"=553197.0}, {"X"=76.95, "Y"=552292.0}, {"X"=77.0, "Y"=551398.0}, {"X"=77.05000000000001, "Y"=550498.0}, {"X"=77.10000000000001, "Y"=549568.0}, {"X"=77.15, "Y"=548647.0}, {"X"=77.2, "Y"=547776.0}, {"X"=77.25, "Y"=546903.0}, {"X"=77.30000000000001, "Y"=545977.0}, {"X"=77.35000000000001, "Y"=545038.0}, {"X"=77.4, "Y"=544131.0}, {"X"=77.45, "Y"=543242.0}, {"X"=77.5, "Y"=542303.0}, {"X"=77.55000000000001, "Y"=541319.0}, {"X"=77.60000000000001, "Y"=540382.0}, {"X"=77.65, "Y"=539547.0}, {"X"=77.7, "Y"=538766.0}, {"X"=77.75, "Y"=537943.0}, {"X"=77.80000000000001, "Y"=537074.0}, {"X"=77.85000000000001, "Y"=536201.0}, {"X"=77.9, "Y"=535266.0}, {"X"=77.95, "Y"=534206.0}, {"X"=78.0, "Y"=533082.0}, {"X"=78.05000000000001, "Y"=532013.0}, {"X"=78.10000000000001, "Y"=531068.0}, {"X"=78.15, "Y"=530258.0}, {"X"=78.2, "Y"=529508.0}, {"X"=78.25, "Y"=528736.0}, {"X"=78.30000000000001, "Y"=527932.0}, {"X"=78.35000000000001, "Y"=527137.0}, {"X"=78.4, "Y"=526307.0}, {"X"=78.45, "Y"=525377.0}, {"X"=78.5, "Y"=524366.0}, {"X"=78.55000000000001, "Y"=523316.0}, {"X"=78.60000000000001, "Y"=522305.0}, {"X"=78.65, "Y"=521431.0}, {"X"=78.7, "Y"=520671.0}, {"X"=78.75, "Y"=519912.0}, {"X"=78.80000000000001, "Y"=519099.0}, {"X"=78.85000000000001, "Y"=518270.0}, {"X"=78.9, "Y"=517425.0}, {"X"=78.95, "Y"=516496.0}, {"X"=79.0, "Y"=515508.0}, {"X"=79.05000000000001, "Y"=514571.0}, {"X"=79.10000000000001, "Y"=513687.0}, {"X"=79.15, "Y"=512772.0}, {"X"=79.2, "Y"=511832.0}, {"X"=79.25, "Y"=510897.0}, {"X"=79.30000000000001, "Y"=509983.0}, {"X"=79.35000000000001, "Y"=509140.0}, {"X"=79.4, "Y"=508358.0}, {"X"=79.45, "Y"=507530.0}, {"X"=79.5, "Y"=506584.0}, {"X"=79.55000000000001, "Y"=505585.0}, {"X"=79.60000000000001, "Y"=504696.0}, {"X"=79.65, "Y"=503894.0}, {"X"=79.7, "Y"=502969.0}, {"X"=79.75, "Y"=501920.0}, {"X"=79.80000000000001, "Y"=501013.0}, {"X"=79.85000000000001, "Y"=500331.0}, {"X"=79.9, "Y"=499657.0}, {"X"=79.95, "Y"=498889.0}, {"X"=80.0, "Y"=498137.0}, {"X"=80.05000000000001, "Y"=497427.0}, {"X"=80.10000000000001, "Y"=496626.0}, {"X"=80.15, "Y"=495661.0}, {"X"=80.2, "Y"=494610.0}, {"X"=80.25, "Y"=493555.0}, {"X"=80.30000000000001, "Y"=492506.0}, {"X"=80.35000000000001, "Y"=491513.0}, {"X"=80.4, "Y"=490654.0}, {"X"=80.45, "Y"=489885.0}, {"X"=80.5, "Y"=489074.0}, {"X"=80.55000000000001, "Y"=488172.0}, {"X"=80.60000000000001, "Y"=487278.0}, {"X"=80.65, "Y"=486477.0}, {"X"=80.7, "Y"=485687.0}, {"X"=80.75, "Y"=484835.0}, {"X"=80.80000000000001, "Y"=483989.0}, {"X"=80.85000000000001, "Y"=483215.0}, {"X"=80.9, "Y"=482458.0}, {"X"=80.95, "Y"=481637.0}, {"X"=81.0, "Y"=480732.0}, {"X"=81.05000000000001, "Y"=479752.0}, {"X"=81.10000000000001, "Y"=478794.0}, {"X"=81.15, "Y"=477990.0}, {"X"=81.2, "Y"=477312.0}, {"X"=81.25, "Y"=476649.0}, {"X"=81.30000000000001, "Y"=475858.0}, {"X"=81.35000000000001, "Y"=474894.0}, {"X"=81.4, "Y"=473909.0}, {"X"=81.45, "Y"=473032.0}, {"X"=81.5, "Y"=472245.0}, {"X"=81.55000000000001, "Y"=471457.0}, {"X"=81.60000000000001, "Y"=470557.0}, {"X"=81.65, "Y"=469593.0}, {"X"=81.7, "Y"=468705.0}, {"X"=81.75, "Y"=467935.0}, {"X"=81.80000000000001, "Y"=467235.0}, {"X"=81.85000000000001, "Y"=466548.0}, {"X"=81.9, "Y"=465854.0}, {"X"=81.95, "Y"=465189.0}, {"X"=82.0, "Y"=464525.0}, {"X"=82.05000000000001, "Y"=463808.0}, {"X"=82.10000000000001, "Y"=463052.0}, {"X"=82.15, "Y"=462311.0}, {"X"=82.2, "Y"=461572.0}, {"X"=82.25, "Y"=460767.0}, {"X"=82.30000000000001, "Y"=459872.0}, {"X"=82.35000000000001, "Y"=458978.0}, {"X"=82.4, "Y"=458160.0}, {"X"=82.45, "Y"=457357.0}, {"X"=82.5, "Y"=456464.0}, {"X"=82.55000000000001, "Y"=455538.0}, {"X"=82.60000000000001, "Y"=454688.0}, {"X"=82.65, "Y"=453895.0}, {"X"=82.7, "Y"=453080.0}, {"X"=82.75, "Y"=452272.0}, {"X"=82.80000000000001, "Y"=451506.0}, {"X"=82.85000000000001, "Y"=450713.0}, {"X"=82.9, "Y"=449849.0}, {"X"=82.95, "Y"=449007.0}, {"X"=83.0, "Y"=448232.0}, {"X"=83.05000000000001, "Y"=447503.0}, {"X"=83.10000000000001, "Y"=446781.0}, {"X"=83.15, "Y"=446002.0}, {"X"=83.2, "Y"=445190.0}, {"X"=83.25, "Y"=444444.0}, {"X"=83.30000000000001, "Y"=443773.0}, {"X"=83.35000000000001, "Y"=443083.0}, {"X"=83.4, "Y"=442322.0}, {"X"=83.45, "Y"=441515.0}, {"X"=83.5, "Y"=440689.0}, {"X"=83.55000000000001, "Y"=439827.0}, {"X"=83.60000000000001, "Y"=438949.0}, {"X"=83.65, "Y"=438135.0}, {"X"=83.7, "Y"=437441.0}, {"X"=83.75, "Y"=436840.0}, {"X"=83.80000000000001, "Y"=436259.0}, {"X"=83.85000000000001, "Y"=435642.0}, {"X"=83.9, "Y"=434928.0}, {"X"=83.95, "Y"=434128.0}, {"X"=84.0, "Y"=433280.0}, {"X"=84.05000000000001, "Y"=432399.0}, {"X"=84.10000000000001, "Y"=431550.0}, {"X"=84.15, "Y"=430799.0}, {"X"=84.2, "Y"=430115.0}, {"X"=84.25, "Y"=429439.0}, {"X"=84.30000000000001, "Y"=428725.0}, {"X"=84.35000000000001, "Y"=427977.0}, {"X"=84.4, "Y"=427242.0}, {"X"=84.45, "Y"=426557.0}, {"X"=84.5, "Y"=425852.0}, {"X"=84.55000000000001, "Y"=425029.0}, {"X"=84.60000000000001, "Y"=424152.0}, {"X"=84.65, "Y"=423362.0}, {"X"=84.7, "Y"=422689.0}, {"X"=84.75, "Y"=422043.0}, {"X"=84.80000000000001, "Y"=421378.0}, {"X"=84.85000000000001, "Y"=420718.0}, {"X"=84.9, "Y"=420069.0}, {"X"=84.95, "Y"=419429.0}, {"X"=85.0, "Y"=418785.0}, {"X"=85.05000000000001, "Y"=418132.0}, {"X"=85.10000000000001, "Y"=417491.0}, {"X"=85.15, "Y"=416853.0}, {"X"=85.2, "Y"=416167.0}, {"X"=85.25, "Y"=415435.0}, {"X"=85.30000000000001, "Y"=414736.0}, {"X"=85.35000000000001, "Y"=414130.0}, {"X"=85.4, "Y"=413574.0}, {"X"=85.45, "Y"=412968.0}, {"X"=85.5, "Y"=412280.0}, {"X"=85.55000000000001, "Y"=411570.0}, {"X"=85.60000000000001, "Y"=410876.0}, {"X"=85.65, "Y"=410167.0}, {"X"=85.7, "Y"=409395.0}, {"X"=85.75, "Y"=408585.0}, {"X"=85.80000000000001, "Y"=407829.0}, {"X"=85.85000000000001, "Y"=407163.0}, {"X"=85.9, "Y"=406540.0}, {"X"=85.95, "Y"=405920.0}, {"X"=86.0, "Y"=405273.0}, {"X"=86.05000000000001, "Y"=404588.0}, {"X"=86.10000000000001, "Y"=403908.0}, {"X"=86.15, "Y"=403271.0}, {"X"=86.2, "Y"=402664.0}, {"X"=86.25, "Y"=402057.0}, {"X"=86.30000000000001, "Y"=401469.0}, {"X"=86.35000000000001, "Y"=400881.0}, {"X"=86.4, "Y"=400247.0}, {"X"=86.45, "Y"=399631.0}, {"X"=86.5, "Y"=399083.0}, {"X"=86.55000000000001, "Y"=398513.0}, {"X"=86.60000000000001, "Y"=397851.0}, {"X"=86.65, "Y"=397183.0}, {"X"=86.7, "Y"=396629.0}, {"X"=86.75, "Y"=396139.0}, {"X"=86.80000000000001, "Y"=395576.0}, {"X"=86.85000000000001, "Y"=394927.0}, {"X"=86.9, "Y"=394304.0}, {"X"=86.95, "Y"=393749.0}, {"X"=87.0, "Y"=393182.0}, {"X"=87.05000000000001, "Y"=392551.0}, {"X"=87.10000000000001, "Y"=391894.0}, {"X"=87.15, "Y"=391224.0}, {"X"=87.2, "Y"=390529.0}, {"X"=87.25, "Y"=389862.0}, {"X"=87.30000000000001, "Y"=389268.0}, {"X"=87.35000000000001, "Y"=388695.0}, {"X"=87.4, "Y"=388112.0}, {"X"=87.45, "Y"=387519.0}, {"X"=87.5, "Y"=386935.0}, {"X"=87.55000000000001, "Y"=386367.0}, {"X"=87.60000000000001, "Y"=385790.0}, {"X"=87.65, "Y"=385244.0}, {"X"=87.7, "Y"=384784.0}, {"X"=87.75, "Y"=384340.0}, {"X"=87.80000000000001, "Y"=383799.0}, {"X"=87.85000000000001, "Y"=383171.0}, {"X"=87.9, "Y"=382528.0}, {"X"=87.95, "Y"=381899.0}, {"X"=88.0, "Y"=381265.0}, {"X"=88.05000000000001, "Y"=380640.0}, {"X"=88.10000000000001, "Y"=380050.0}, {"X"=88.15, "Y"=379471.0}, {"X"=88.2, "Y"=378870.0}, {"X"=88.25, "Y"=378270.0}, {"X"=88.30000000000001, "Y"=377710.0}, {"X"=88.35000000000001, "Y"=377177.0}, {"X"=88.4, "Y"=376616.0}, {"X"=88.45, "Y"=376014.0}, {"X"=88.5, "Y"=375406.0}, {"X"=88.55000000000001, "Y"=374846.0}, {"X"=88.60000000000001, "Y"=374295.0}, {"X"=88.65, "Y"=373640.0}, {"X"=88.7, "Y"=372935.0}, {"X"=88.75, "Y"=372316.0}, {"X"=88.80000000000001, "Y"=371735.0}, {"X"=88.85000000000001, "Y"=371106.0}, {"X"=88.9, "Y"=370503.0}, {"X"=88.95, "Y"=369974.0}, {"X"=89.0, "Y"=369451.0}, {"X"=89.05000000000001, "Y"=368885.0}, {"X"=89.10000000000001, "Y"=368306.0}, {"X"=89.15, "Y"=367752.0}, {"X"=89.2, "Y"=367204.0}, {"X"=89.25, "Y"=366615.0}, {"X"=89.30000000000001, "Y"=366031.0}, {"X"=89.35000000000001, "Y"=365497.0}, {"X"=89.4, "Y"=364972.0}, {"X"=89.45, "Y"=364398.0}, {"X"=89.5, "Y"=363771.0}, {"X"=89.55000000000001, "Y"=363137.0}, {"X"=89.60000000000001, "Y"=362550.0}, {"X"=89.65, "Y"=362033.0}, {"X"=89.7, "Y"=361546.0}, {"X"=89.75, "Y"=361029.0}, {"X"=89.80000000000001, "Y"=360466.0}, {"X"=89.85000000000001, "Y"=359909.0}, {"X"=89.9, "Y"=359388.0}, {"X"=89.95, "Y"=358873.0}, {"X"=90.0, "Y"=358348.0}, {"X"=90.05000000000001, "Y"=357842.0}, {"X"=90.10000000000001, "Y"=357364.0}, {"X"=90.15, "Y"=356876.0}, {"X"=90.2, "Y"=356318.0}, {"X"=90.25, "Y"=355688.0}, {"X"=90.30000000000001, "Y"=355084.0}, {"X"=90.35000000000001, "Y"=354569.0}, {"X"=90.4, "Y"=354106.0}, {"X"=90.45, "Y"=353636.0}, {"X"=90.5, "Y"=353145.0}, {"X"=90.55000000000001, "Y"=352632.0}, {"X"=90.60000000000001, "Y"=352100.0}, {"X"=90.65, "Y"=351528.0}, {"X"=90.7, "Y"=350923.0}, {"X"=90.75, "Y"=350340.0}, {"X"=90.80000000000001, "Y"=349800.0}, {"X"=90.85000000000001, "Y"=349309.0}, {"X"=90.9, "Y"=348812.0}, {"X"=90.95, "Y"=348237.0}, {"X"=91.0, "Y"=347627.0}, {"X"=91.05000000000001, "Y"=347080.0}, {"X"=91.10000000000001, "Y"=346641.0}, {"X"=91.15, "Y"=346275.0}, {"X"=91.2, "Y"=345912.0}, {"X"=91.25, "Y"=345518.0}, {"X"=91.30000000000001, "Y"=345092.0}, {"X"=91.35000000000001, "Y"=344634.0}, {"X"=91.4, "Y"=344114.0}, {"X"=91.45, "Y"=343521.0}, {"X"=91.5, "Y"=342879.0}, {"X"=91.55000000000001, "Y"=342225.0}, {"X"=91.60000000000001, "Y"=341619.0}, {"X"=91.65, "Y"=341084.0}, {"X"=91.7, "Y"=340557.0}, {"X"=91.75, "Y"=340007.0}, {"X"=91.80000000000001, "Y"=339506.0}, {"X"=91.85000000000001, "Y"=339089.0}, {"X"=91.9, "Y"=338666.0}, {"X"=91.95, "Y"=338204.0}, {"X"=92.0, "Y"=337759.0}, {"X"=92.05000000000001, "Y"=337310.0}, {"X"=92.10000000000001, "Y"=336798.0}, {"X"=92.15, "Y"=336261.0}, {"X"=92.2, "Y"=335766.0}, {"X"=92.25, "Y"=335302.0}, {"X"=92.30000000000001, "Y"=334827.0}, {"X"=92.35000000000001, "Y"=334340.0}, {"X"=92.4, "Y"=333871.0}, {"X"=92.45, "Y"=333422.0}, {"X"=92.5, "Y"=332957.0}, {"X"=92.55000000000001, "Y"=332481.0}, {"X"=92.60000000000001, "Y"=332023.0}, {"X"=92.65, "Y"=331588.0}, {"X"=92.7, "Y"=331123.0}, {"X"=92.75, "Y"=330619.0}, {"X"=92.80000000000001, "Y"=330120.0}, {"X"=92.85000000000001, "Y"=329665.0}, {"X"=92.9, "Y"=329228.0}, {"X"=92.95, "Y"=328734.0}, {"X"=93.0, "Y"=328191.0}, {"X"=93.05000000000001, "Y"=327666.0}, {"X"=93.10000000000001, "Y"=327164.0}, {"X"=93.15, "Y"=326667.0}, {"X"=93.2, "Y"=326190.0}, {"X"=93.25, "Y"=325754.0}, {"X"=93.30000000000001, "Y"=325326.0}, {"X"=93.35000000000001, "Y"=324864.0}, {"X"=93.4, "Y"=324371.0}, {"X"=93.45, "Y"=323873.0}, {"X"=93.5, "Y"=323427.0}, {"X"=93.55000000000001, "Y"=323079.0}, {"X"=93.60000000000001, "Y"=322754.0}, {"X"=93.65, "Y"=322337.0}, {"X"=93.7, "Y"=321823.0}, {"X"=93.75, "Y"=321301.0}, {"X"=93.80000000000001, "Y"=320799.0}, {"X"=93.85000000000001, "Y"=320296.0}, {"X"=93.9, "Y"=319838.0}, {"X"=93.95, "Y"=319462.0}, {"X"=94.0, "Y"=319096.0}, {"X"=94.05000000000001, "Y"=318689.0}, {"X"=94.10000000000001, "Y"=318291.0}, {"X"=94.15, "Y"=317942.0}, {"X"=94.2, "Y"=317591.0}, {"X"=94.25, "Y"=317186.0}, {"X"=94.30000000000001, "Y"=316751.0}, {"X"=94.35000000000001, "Y"=316339.0}, {"X"=94.4, "Y"=315960.0}, {"X"=94.45, "Y"=315586.0}, {"X"=94.5, "Y"=315194.0}, {"X"=94.55000000000001, "Y"=314808.0}, {"X"=94.60000000000001, "Y"=314450.0}, {"X"=94.65, "Y"=314091.0}, {"X"=94.7, "Y"=313712.0}, {"X"=94.75, "Y"=313325.0}, {"X"=94.80000000000001, "Y"=312956.0}, {"X"=94.85000000000001, "Y"=312614.0}, {"X"=94.9, "Y"=312257.0}, {"X"=94.95, "Y"=311824.0}, {"X"=95.0, "Y"=311333.0}, {"X"=95.05000000000001, "Y"=310848.0}, {"X"=95.10000000000001, "Y"=310403.0}, {"X"=95.15, "Y"=310009.0}, {"X"=95.2, "Y"=309678.0}, {"X"=95.25, "Y"=309386.0}, {"X"=95.30000000000001, "Y"=309091.0}, {"X"=95.35000000000001, "Y"=308758.0}, {"X"=95.4, "Y"=308387.0}, {"X"=95.45, "Y"=307975.0}, {"X"=95.5, "Y"=307490.0}, {"X"=95.55000000000001, "Y"=307004.0}, {"X"=95.60000000000001, "Y"=306615.0}, {"X"=95.65, "Y"=306290.0}, {"X"=95.7, "Y"=305952.0}, {"X"=95.75, "Y"=305547.0}, {"X"=95.80000000000001, "Y"=305072.0}, {"X"=95.85000000000001, "Y"=304593.0}, {"X"=95.9, "Y"=304170.0}, {"X"=95.95, "Y"=303835.0}, {"X"=96.0, "Y"=303533.0}, {"X"=96.05000000000001, "Y"=303198.0}, {"X"=96.10000000000001, "Y"=302846.0}, {"X"=96.15, "Y"=302479.0}, {"X"=96.2, "Y"=302092.0}, {"X"=96.25, "Y"=301677.0}, {"X"=96.30000000000001, "Y"=301235.0}, {"X"=96.35000000000001, "Y"=300795.0}, {"X"=96.4, "Y"=300390.0}, {"X"=96.45, "Y"=300019.0}, {"X"=96.5, "Y"=299666.0}, {"X"=96.55000000000001, "Y"=299296.0}, {"X"=96.60000000000001, "Y"=298912.0}, {"X"=96.65, "Y"=298563.0}, {"X"=96.7, "Y"=298238.0}, {"X"=96.75, "Y"=297872.0}, {"X"=96.80000000000001, "Y"=297465.0}, {"X"=96.85000000000001, "Y"=297080.0}, {"X"=96.9, "Y"=296750.0}, {"X"=96.95, "Y"=296435.0}, {"X"=97.0, "Y"=296093.0}, {"X"=97.05000000000001, "Y"=295740.0}, {"X"=97.10000000000001, "Y"=295398.0}, {"X"=97.15, "Y"=295044.0}, {"X"=97.2, "Y"=294654.0}, {"X"=97.25, "Y"=294210.0}, {"X"=97.30000000000001, "Y"=293728.0}, {"X"=97.35000000000001, "Y"=293261.0}, {"X"=97.4, "Y"=292846.0}, {"X"=97.45, "Y"=292460.0}, {"X"=97.5, "Y"=292058.0}, {"X"=97.55000000000001, "Y"=291638.0}, {"X"=97.60000000000001, "Y"=291252.0}, {"X"=97.65, "Y"=290913.0}, {"X"=97.7, "Y"=290572.0}, {"X"=97.75, "Y"=290231.0}, {"X"=97.80000000000001, "Y"=289902.0}, {"X"=97.85000000000001, "Y"=289567.0}, {"X"=97.9, "Y"=289205.0}, {"X"=97.95, "Y"=288849.0}, {"X"=98.0, "Y"=288531.0}, {"X"=98.05000000000001, "Y"=288224.0}, {"X"=98.10000000000001, "Y"=287904.0}, {"X"=98.15, "Y"=287552.0}, {"X"=98.2, "Y"=287166.0}, {"X"=98.25, "Y"=286809.0}, {"X"=98.30000000000001, "Y"=286497.0}, {"X"=98.35000000000001, "Y"=286172.0}, {"X"=98.4, "Y"=285813.0}, {"X"=98.45, "Y"=285458.0}, {"X"=98.5, "Y"=285103.0}, {"X"=98.55000000000001, "Y"=284728.0}, {"X"=98.60000000000001, "Y"=284324.0}, {"X"=98.65, "Y"=283859.0}, {"X"=98.7, "Y"=283391.0}, {"X"=98.75, "Y"=283040.0}, {"X"=98.80000000000001, "Y"=282808.0}, {"X"=98.85000000000001, "Y"=282609.0}, {"X"=98.9, "Y"=282373.0}, {"X"=98.95, "Y"=282113.0}, {"X"=99.0, "Y"=281866.0}, {"X"=99.05000000000001, "Y"=281633.0}, {"X"=99.10000000000001, "Y"=281394.0}, {"X"=99.15, "Y"=281076.0}, {"X"=99.2, "Y"=280635.0}, {"X"=99.25, "Y"=280141.0}, {"X"=99.30000000000001, "Y"=279690.0}, {"X"=99.35000000000001, "Y"=279326.0}, {"X"=99.4, "Y"=279013.0}, {"X"=99.45, "Y"=278673.0}, {"X"=99.5, "Y"=278319.0}, {"X"=99.55000000000001, "Y"=278020.0}, {"X"=99.60000000000001, "Y"=277722.0}, {"X"=99.65, "Y"=277350.0}, {"X"=99.7, "Y"=276964.0}, {"X"=99.75, "Y"=276641.0}, {"X"=99.80000000000001, "Y"=276381.0}, {"X"=99.85000000000001, "Y"=276109.0}, {"X"=99.9, "Y"=275801.0}, {"X"=99.95, "Y"=275484.0}, {"X"=100.0, "Y"=275157.0}, {"X"=100.05000000000001, "Y"=274790.0}, {"X"=100.10000000000001, "Y"=274397.0}, {"X"=100.15, "Y"=274037.0}, {"X"=100.2, "Y"=273755.0}, {"X"=100.25, "Y"=273507.0}, {"X"=100.30000000000001, "Y"=273250.0}, {"X"=100.35000000000001, "Y"=272967.0}, {"X"=100.4, "Y"=272655.0}, {"X"=100.45, "Y"=272344.0}, {"X"=100.5, "Y"=272037.0}, {"X"=100.55000000000001, "Y"=271702.0}, {"X"=100.60000000000001, "Y"=271329.0}, {"X"=100.65, "Y"=270945.0}, {"X"=100.7, "Y"=270589.0}, {"X"=100.75, "Y"=270291.0}, {"X"=100.80000000000001, "Y"=270000.0}, {"X"=100.85000000000001, "Y"=269664.0}, {"X"=100.9, "Y"=269305.0}, {"X"=100.95, "Y"=268978.0}, {"X"=101.0, "Y"=268688.0}, {"X"=101.05000000000001, "Y"=268414.0}, {"X"=101.10000000000001, "Y"=268131.0}, {"X"=101.15, "Y"=267841.0}, {"X"=101.2, "Y"=267522.0}, {"X"=101.25, "Y"=267144.0}, {"X"=101.30000000000001, "Y"=266728.0}, {"X"=101.35000000000001, "Y"=266342.0}, {"X"=101.4, "Y"=266040.0}, {"X"=101.45, "Y"=265788.0}, {"X"=101.5, "Y"=265514.0}, {"X"=101.55000000000001, "Y"=265197.0}, {"X"=101.60000000000001, "Y"=264866.0}, {"X"=101.65, "Y"=264535.0}, {"X"=101.7, "Y"=264187.0}, {"X"=101.75, "Y"=263810.0}, {"X"=101.80000000000001, "Y"=263404.0}, {"X"=101.85000000000001, "Y"=262976.0}, {"X"=101.9, "Y"=262576.0}, {"X"=101.95, "Y"=262250.0}, {"X"=102.0, "Y"=261960.0}, {"X"=102.05000000000001, "Y"=261676.0}, {"X"=102.10000000000001, "Y"=261429.0}, {"X"=102.15, "Y"=261217.0}, {"X"=102.2, "Y"=260977.0}, {"X"=102.25, "Y"=260683.0}, {"X"=102.30000000000001, "Y"=260367.0}, {"X"=102.35000000000001, "Y"=260051.0}, {"X"=102.4, "Y"=259728.0}, {"X"=102.45, "Y"=259402.0}, {"X"=102.5, "Y"=259084.0}, {"X"=102.55000000000001, "Y"=258770.0}, {"X"=102.60000000000001, "Y"=258459.0}, {"X"=102.65, "Y"=258184.0}, {"X"=102.7, "Y"=257931.0}, {"X"=102.75, "Y"=257652.0}, {"X"=102.80000000000001, "Y"=257340.0}, {"X"=102.85000000000001, "Y"=257016.0}, {"X"=102.9, "Y"=256709.0}, {"X"=102.95, "Y"=256411.0}, {"X"=103.0, "Y"=256095.0}, {"X"=103.05000000000001, "Y"=255770.0}, {"X"=103.10000000000001, "Y"=255463.0}, {"X"=103.15, "Y"=255147.0}, {"X"=103.2, "Y"=254807.0}, {"X"=103.25, "Y"=254468.0}, {"X"=103.30000000000001, "Y"=254129.0}, {"X"=103.35000000000001, "Y"=253783.0}, {"X"=103.4, "Y"=253430.0}, {"X"=103.45, "Y"=253095.0}, {"X"=103.5, "Y"=252792.0}, {"X"=103.55000000000001, "Y"=252496.0}, {"X"=103.60000000000001, "Y"=252213.0}, {"X"=103.65, "Y"=251939.0}, {"X"=103.7, "Y"=251665.0}, {"X"=103.75, "Y"=251400.0}, {"X"=103.80000000000001, "Y"=251121.0}, {"X"=103.85000000000001, "Y"=250811.0}, {"X"=103.9, "Y"=250513.0}, {"X"=103.95, "Y"=250249.0}, {"X"=104.0, "Y"=249978.0}, {"X"=104.05000000000001, "Y"=249684.0}, {"X"=104.10000000000001, "Y"=249408.0}, {"X"=104.15, "Y"=249168.0}, {"X"=104.2, "Y"=248920.0}, {"X"=104.25, "Y"=248635.0}, {"X"=104.30000000000001, "Y"=248344.0}, {"X"=104.35000000000001, "Y"=248062.0}, {"X"=104.4, "Y"=247754.0}, {"X"=104.45, "Y"=247393.0}, {"X"=104.5, "Y"=247028.0}, {"X"=104.55000000000001, "Y"=246712.0}, {"X"=104.60000000000001, "Y"=246431.0}, {"X"=104.65, "Y"=246138.0}, {"X"=104.7, "Y"=245835.0}, {"X"=104.75, "Y"=245574.0}, {"X"=104.80000000000001, "Y"=245364.0}, {"X"=104.85000000000001, "Y"=245155.0}, {"X"=104.9, "Y"=244906.0}, {"X"=104.95, "Y"=244633.0}, {"X"=105.0, "Y"=244350.0}, {"X"=105.05000000000001, "Y"=244044.0}, {"X"=105.10000000000001, "Y"=243726.0}, {"X"=105.15, "Y"=243420.0}, {"X"=105.2, "Y"=243111.0}, {"X"=105.25, "Y"=242787.0}, {"X"=105.30000000000001, "Y"=242451.0}, {"X"=105.35000000000001, "Y"=242106.0}, {"X"=105.4, "Y"=241753.0}, {"X"=105.45, "Y"=241428.0}, {"X"=105.5, "Y"=241142.0}, {"X"=105.55000000000001, "Y"=240872.0}, {"X"=105.60000000000001, "Y"=240627.0}, {"X"=105.65, "Y"=240409.0}, {"X"=105.7, "Y"=240173.0}, {"X"=105.75, "Y"=239904.0}, {"X"=105.80000000000001, "Y"=239623.0}, {"X"=105.85000000000001, "Y"=239325.0}, {"X"=105.9, "Y"=238998.0}, {"X"=105.95, "Y"=238659.0}, {"X"=106.0, "Y"=238359.0}, {"X"=106.05000000000001, "Y"=238106.0}, {"X"=106.10000000000001, "Y"=237850.0}, {"X"=106.15, "Y"=237562.0}, {"X"=106.2, "Y"=237270.0}, {"X"=106.25, "Y"=237006.0}, {"X"=106.30000000000001, "Y"=236756.0}, {"X"=106.35000000000001, "Y"=236471.0}, {"X"=106.4, "Y"=236140.0}, {"X"=106.45, "Y"=235794.0}, {"X"=106.5, "Y"=235467.0}, {"X"=106.55000000000001, "Y"=235158.0}, {"X"=106.60000000000001, "Y"=234832.0}, {"X"=106.65, "Y"=234497.0}, {"X"=106.7, "Y"=234231.0}, {"X"=106.75, "Y"=234056.0}, {"X"=106.80000000000001, "Y"=233899.0}, {"X"=106.85000000000001, "Y"=233686.0}, {"X"=106.9, "Y"=233428.0}, {"X"=106.95, "Y"=233177.0}, {"X"=107.0, "Y"=232954.0}, {"X"=107.05000000000001, "Y"=232709.0}, {"X"=107.10000000000001, "Y"=232410.0}, {"X"=107.15, "Y"=232097.0}, {"X"=107.2, "Y"=231817.0}, {"X"=107.25, "Y"=231568.0}, {"X"=107.30000000000001, "Y"=231322.0}, {"X"=107.35000000000001, "Y"=231047.0}, {"X"=107.4, "Y"=230739.0}, {"X"=107.45, "Y"=230414.0}, {"X"=107.5, "Y"=230106.0}, {"X"=107.55000000000001, "Y"=229810.0}, {"X"=107.60000000000001, "Y"=229497.0}, {"X"=107.65, "Y"=229178.0}, {"X"=107.7, "Y"=228884.0}, {"X"=107.75, "Y"=228625.0}, {"X"=107.80000000000001, "Y"=228391.0}, {"X"=107.85000000000001, "Y"=228147.0}, {"X"=107.9, "Y"=227900.0}, {"X"=107.95, "Y"=227666.0}, {"X"=108.0, "Y"=227435.0}, {"X"=108.05000000000001, "Y"=227236.0}, {"X"=108.10000000000001, "Y"=227098.0}, {"X"=108.15, "Y"=226948.0}, {"X"=108.2, "Y"=226699.0}, {"X"=108.25, "Y"=226407.0}, {"X"=108.30000000000001, "Y"=226143.0}, {"X"=108.35000000000001, "Y"=225888.0}, {"X"=108.4, "Y"=225583.0}, {"X"=108.45, "Y"=225257.0}, {"X"=108.5, "Y"=224952.0}, {"X"=108.55000000000001, "Y"=224659.0}, {"X"=108.60000000000001, "Y"=224406.0}, {"X"=108.65, "Y"=224165.0}, {"X"=108.7, "Y"=223892.0}, {"X"=108.75, "Y"=223623.0}, {"X"=108.80000000000001, "Y"=223376.0}, {"X"=108.85000000000001, "Y"=223139.0}, {"X"=108.9, "Y"=222880.0}, {"X"=108.95, "Y"=222591.0}, {"X"=109.0, "Y"=222343.0}, {"X"=109.05000000000001, "Y"=222172.0}, {"X"=109.10000000000001, "Y"=222034.0}, {"X"=109.15, "Y"=221891.0}, {"X"=109.2, "Y"=221734.0}, {"X"=109.25, "Y"=221553.0}, {"X"=109.30000000000001, "Y"=221344.0}, {"X"=109.35000000000001, "Y"=221079.0}, {"X"=109.4, "Y"=220746.0}, {"X"=109.45, "Y"=220389.0}, {"X"=109.5, "Y"=220080.0}, {"X"=109.55000000000001, "Y"=219818.0}, {"X"=109.60000000000001, "Y"=219557.0}, {"X"=109.65, "Y"=219295.0}, {"X"=109.7, "Y"=219048.0}, {"X"=109.75, "Y"=218793.0}, {"X"=109.80000000000001, "Y"=218517.0}, {"X"=109.85000000000001, "Y"=218242.0}, {"X"=109.9, "Y"=217997.0}, {"X"=109.95, "Y"=217784.0}, {"X"=110.0, "Y"=217585.0}, {"X"=110.05000000000001, "Y"=217403.0}, {"X"=110.10000000000001, "Y"=217242.0}, {"X"=110.15, "Y"=217083.0}, {"X"=110.2, "Y"=216913.0}, {"X"=110.25, "Y"=216734.0}, {"X"=110.30000000000001, "Y"=216547.0}, {"X"=110.35000000000001, "Y"=216345.0}, {"X"=110.4, "Y"=216116.0}, {"X"=110.45, "Y"=215870.0}, {"X"=110.5, "Y"=215662.0}, {"X"=110.55000000000001, "Y"=215498.0}, {"X"=110.60000000000001, "Y"=215336.0}, {"X"=110.65, "Y"=215141.0}, {"X"=110.7, "Y"=214907.0}, {"X"=110.75, "Y"=214650.0}, {"X"=110.80000000000001, "Y"=214375.0}, {"X"=110.85000000000001, "Y"=214058.0}, {"X"=110.9, "Y"=213728.0}, {"X"=110.95, "Y"=213463.0}, {"X"=111.0, "Y"=213245.0}, {"X"=111.05000000000001, "Y"=213018.0}, {"X"=111.10000000000001, "Y"=212801.0}, {"X"=111.15, "Y"=212624.0}, {"X"=111.2, "Y"=212451.0}, {"X"=111.25, "Y"=212251.0}, {"X"=111.30000000000001, "Y"=212046.0}, {"X"=111.35000000000001, "Y"=211856.0}, {"X"=111.4, "Y"=211652.0}, {"X"=111.45, "Y"=211395.0}, {"X"=111.5, "Y"=211112.0}, {"X"=111.55000000000001, "Y"=210864.0}, {"X"=111.60000000000001, "Y"=210683.0}, {"X"=111.65, "Y"=210550.0}, {"X"=111.7, "Y"=210418.0}, {"X"=111.75, "Y"=210250.0}, {"X"=111.80000000000001, "Y"=210044.0}, {"X"=111.85000000000001, "Y"=209819.0}, {"X"=111.9, "Y"=209579.0}, {"X"=111.95, "Y"=209308.0}, {"X"=112.0, "Y"=209017.0}, {"X"=112.05000000000001, "Y"=208720.0}, {"X"=112.10000000000001, "Y"=208453.0}, {"X"=112.15, "Y"=208251.0}, {"X"=112.2, "Y"=208112.0}, {"X"=112.25, "Y"=207982.0}, {"X"=112.30000000000001, "Y"=207831.0}, {"X"=112.35000000000001, "Y"=207675.0}, {"X"=112.4, "Y"=207517.0}, {"X"=112.45, "Y"=207321.0}, {"X"=112.5, "Y"=207106.0}, {"X"=112.55000000000001, "Y"=206913.0}, {"X"=112.60000000000001, "Y"=206743.0}, {"X"=112.65, "Y"=206571.0}, {"X"=112.7, "Y"=206362.0}, {"X"=112.75, "Y"=206142.0}, {"X"=112.80000000000001, "Y"=205962.0}, {"X"=112.85000000000001, "Y"=205772.0}, {"X"=112.9, "Y"=205519.0}, {"X"=112.95, "Y"=205193.0}, {"X"=113.0, "Y"=204835.0}, {"X"=113.05000000000001, "Y"=204548.0}, {"X"=113.10000000000001, "Y"=204364.0}, {"X"=113.15, "Y"=204201.0}, {"X"=113.2, "Y"=204009.0}, {"X"=113.25, "Y"=203800.0}, {"X"=113.30000000000001, "Y"=203585.0}, {"X"=113.35000000000001, "Y"=203381.0}, {"X"=113.4, "Y"=203181.0}, {"X"=113.45, "Y"=202983.0}, {"X"=113.5, "Y"=202796.0}, {"X"=113.55000000000001, "Y"=202612.0}, {"X"=113.60000000000001, "Y"=202420.0}, {"X"=113.65, "Y"=202230.0}, {"X"=113.7, "Y"=202064.0}, {"X"=113.75, "Y"=201907.0}, {"X"=113.80000000000001, "Y"=201719.0}, {"X"=113.85000000000001, "Y"=201497.0}, {"X"=113.9, "Y"=201285.0}, {"X"=113.95, "Y"=201074.0}, {"X"=114.0, "Y"=200847.0}, {"X"=114.05000000000001, "Y"=200618.0}, {"X"=114.10000000000001, "Y"=200382.0}, {"X"=114.15, "Y"=200161.0}, {"X"=114.2, "Y"=200000.0}, {"X"=114.25, "Y"=199869.0}, {"X"=114.30000000000001, "Y"=199721.0}, {"X"=114.35000000000001, "Y"=199561.0}, {"X"=114.4, "Y"=199383.0}, {"X"=114.45, "Y"=199177.0}, {"X"=114.5, "Y"=198971.0}, {"X"=114.55000000000001, "Y"=198792.0}, {"X"=114.60000000000001, "Y"=198617.0}, {"X"=114.65, "Y"=198435.0}, {"X"=114.7, "Y"=198253.0}, {"X"=114.75, "Y"=198065.0}, {"X"=114.80000000000001, "Y"=197893.0}, {"X"=114.85000000000001, "Y"=197751.0}, {"X"=114.9, "Y"=197616.0}, {"X"=114.95, "Y"=197458.0}, {"X"=115.0, "Y"=197274.0}, {"X"=115.05000000000001, "Y"=197071.0}, {"X"=115.10000000000001, "Y"=196846.0}, {"X"=115.15, "Y"=196607.0}, {"X"=115.2, "Y"=196387.0}, {"X"=115.25, "Y"=196168.0}, {"X"=115.30000000000001, "Y"=195928.0}, {"X"=115.35000000000001, "Y"=195686.0}, {"X"=115.4, "Y"=195467.0}, {"X"=115.45, "Y"=195274.0}, {"X"=115.5, "Y"=195088.0}, {"X"=115.55000000000001, "Y"=194897.0}, {"X"=115.60000000000001, "Y"=194708.0}, {"X"=115.65, "Y"=194528.0}, {"X"=115.7, "Y"=194347.0}, {"X"=115.75, "Y"=194157.0}, {"X"=115.80000000000001, "Y"=193967.0}, {"X"=115.85000000000001, "Y"=193789.0}, {"X"=115.9, "Y"=193616.0}, {"X"=115.95, "Y"=193435.0}, {"X"=116.0, "Y"=193257.0}, {"X"=116.05000000000001, "Y"=193086.0}, {"X"=116.10000000000001, "Y"=192899.0}, {"X"=116.15, "Y"=192703.0}, {"X"=116.2, "Y"=192521.0}, {"X"=116.25, "Y"=192341.0}, {"X"=116.30000000000001, "Y"=192136.0}, {"X"=116.35000000000001, "Y"=191915.0}, {"X"=116.4, "Y"=191702.0}, {"X"=116.45, "Y"=191518.0}, {"X"=116.5, "Y"=191361.0}, {"X"=116.55000000000001, "Y"=191214.0}, {"X"=116.60000000000001, "Y"=191053.0}, {"X"=116.65, "Y"=190866.0}, {"X"=116.7, "Y"=190665.0}, {"X"=116.75, "Y"=190473.0}, {"X"=116.80000000000001, "Y"=190298.0}, {"X"=116.85000000000001, "Y"=190129.0}, {"X"=116.9, "Y"=189940.0}, {"X"=116.95, "Y"=189733.0}, {"X"=117.0, "Y"=189541.0}, {"X"=117.05000000000001, "Y"=189365.0}, {"X"=117.10000000000001, "Y"=189205.0}, {"X"=117.15, "Y"=189068.0}, {"X"=117.2, "Y"=188918.0}, {"X"=117.25, "Y"=188721.0}, {"X"=117.30000000000001, "Y"=188488.0}, {"X"=117.35000000000001, "Y"=188246.0}, {"X"=117.4, "Y"=187988.0}, {"X"=117.45, "Y"=187709.0}, {"X"=117.5, "Y"=187452.0}, {"X"=117.55000000000001, "Y"=187223.0}, {"X"=117.60000000000001, "Y"=187016.0}, {"X"=117.65, "Y"=186846.0}, {"X"=117.7, "Y"=186697.0}, {"X"=117.75, "Y"=186530.0}, {"X"=117.80000000000001, "Y"=186373.0}, {"X"=117.85000000000001, "Y"=186241.0}, {"X"=117.9, "Y"=186112.0}, {"X"=117.95, "Y"=185976.0}, {"X"=118.0, "Y"=185829.0}, {"X"=118.05000000000001, "Y"=185656.0}, {"X"=118.10000000000001, "Y"=185476.0}, {"X"=118.15, "Y"=185297.0}, {"X"=118.2, "Y"=185120.0}, {"X"=118.25, "Y"=184960.0}, {"X"=118.30000000000001, "Y"=184802.0}, {"X"=118.35000000000001, "Y"=184626.0}, {"X"=118.4, "Y"=184437.0}, {"X"=118.45, "Y"=184219.0}, {"X"=118.5, "Y"=183973.0}, {"X"=118.55000000000001, "Y"=183747.0}, {"X"=118.60000000000001, "Y"=183568.0}, {"X"=118.65, "Y"=183424.0}, {"X"=118.7, "Y"=183281.0}, {"X"=118.75, "Y"=183122.0}, {"X"=118.80000000000001, "Y"=182948.0}, {"X"=118.85000000000001, "Y"=182777.0}, {"X"=118.9, "Y"=182621.0}, {"X"=118.95, "Y"=182454.0}, {"X"=119.0, "Y"=182244.0}, {"X"=119.05000000000001, "Y"=182039.0}, {"X"=119.10000000000001, "Y"=181901.0}, {"X"=119.15, "Y"=181809.0}, {"X"=119.2, "Y"=181702.0}, {"X"=119.25, "Y"=181560.0}, {"X"=119.30000000000001, "Y"=181429.0}, {"X"=119.35000000000001, "Y"=181330.0}, {"X"=119.4, "Y"=181228.0}, {"X"=119.45, "Y"=181082.0}, {"X"=119.5, "Y"=180905.0}, {"X"=119.55000000000001, "Y"=180730.0}, {"X"=119.60000000000001, "Y"=180549.0}, {"X"=119.65, "Y"=180361.0}, {"X"=119.7, "Y"=180170.0}]}, {[{"X"=18.900000000000002, "Y"=97.0}, {"X"=19.35, "Y"=6644.0}, {"X"=24.950000000000003, "Y"=188.0}, {"X"=25.400000000000002, "Y"=4232.0}, {"X"=27.5, "Y"=15084.0}, {"X"=28.05, "Y"=43.0}, {"X"=38.15, "Y"=5.0}, {"X"=38.650000000000006, "Y"=8382895.0}]}, {[{"X"=19.150000000000002, "Y"=25427.0}, {"X"=19.650000000000002, "Y"=37317.0}, {"X"=25.25, "Y"=8486.0}, {"X"=25.75, "Y"=15898.0}, {"X"=27.8, "Y"=64463573.0}, {"X"=28.400000000000002, "Y"=957.0}, {"X"=38.400000000000006, "Y"=12087206.0}, {"X"=39.0, "Y"=83953263.0}]}, {[{"X"=19.35, "Y"=6644.0}, {"X"=24.950000000000003, "Y"=188.0}, {"X"=25.400000000000002, "Y"=4232.0}, {"X"=27.5, "Y"=15084.0}, {"X"=28.05, "Y"=43.0}, {"X"=31.6, "Y"=74.0}, {"X"=38.650000000000006, "Y"=8382895.0}, {"X"=119.45, "Y"=181082.0}]}, {[{"X"=0.30000000000000004, "Y"=88.0}, {"X"=16.7, "Y"=84.0}, {"X"=18.900000000000002, "Y"=97.0}, {"X"=24.950000000000003, "Y"=188.0}, {"X"=25.0, "Y"=190.0}, {"X"=28.05, "Y"=43.0}, {"X"=28.150000000000002, "Y"=84.0}, {"X"=38.0, "Y"=5.0}, {"X"=38.15, "Y"=5.0}, {"X"=119.45, "Y"=181082.0}]}], 9 "Signal 2":T1=enum."Test Signal", 11 "table in":string[][](table)=[["", "", "", "", "", "", "", ""], ["1", "2", "3", "4", "5", "6", "7", "8"], ["19", "20", "25", "26", "28", "28", "38", "39"], ["3.1101E+3", "8.0538E+4", "1.1111E+3", "1.1949E+4", "1.1887E+7", "8.6898E+2", "1.8080E+6", "1.5851E+8"], ["", "", "", "", "", "", "", ""], ["", "", "", "", "", "", "", ""], ["1", "2", "", "", "", "", "", ""], ["15", "105", "", "", "", "", "", ""], ["1.9635E+5", "1.8829E+5", "", "", "", "", "", ""]]) -> (7 "Det in use":string)   [LabVIEW 2012]
uses:
  signal.ctl
panel:
  in  "Comments":string
  in  "ok":bool
  out "table":string[][](table)=[["", "1", "15"], ["", "2", "105"], ["", "", ""], ["", "", ""], ["", "", ""], ["", "", ""], ["", "", ""], ["", "", ""]]
  in  "box":string
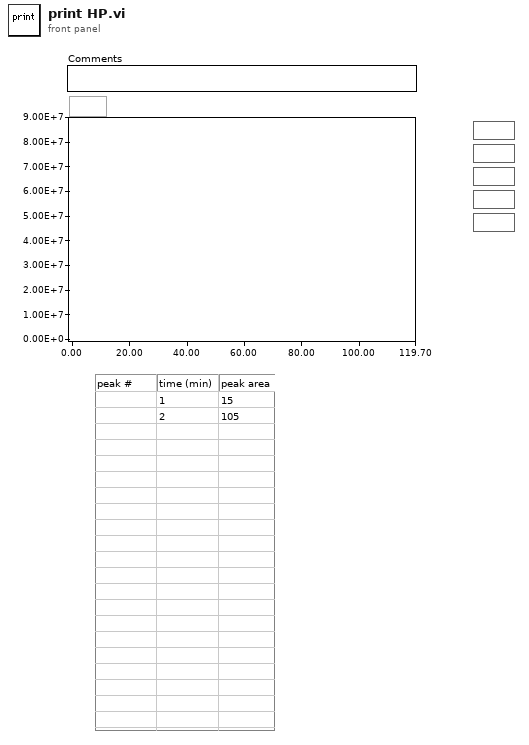
[diagram p1: front panel]
types:
  T1 = typedef "signal.ctl" = enum16{"Detector A", "Detector B", "Oven temperature", "Comp 1", "Comp 2", "Inlet A temperature", "Inlet B temperature", "Detector A temperature", "Detector B temperature", "Test Signal"}
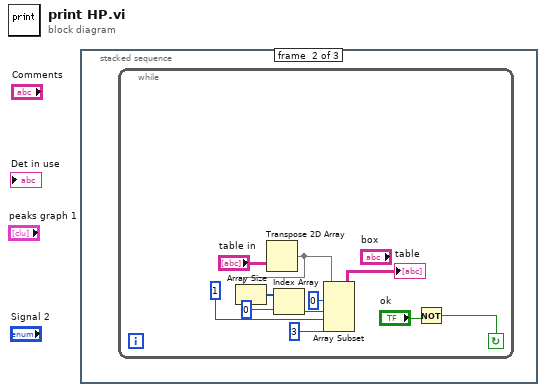
[diagram p0: block diagram]
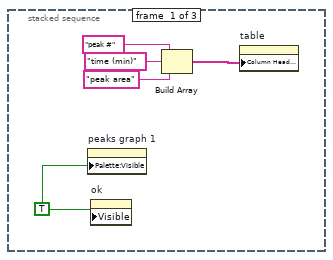
[diagram p2: hidden frame]
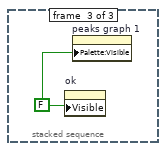
[diagram p3: hidden frame]
diagram:
  n1 = stacked-sequence {
    frame #0 {
      w1 = TRUE
      n2 = property on="peaks graph 1" class="XYGraph (strict)"("Palette:Visible"=w1) -> ()  [unwired: 2 in, 2 out]
      n3 = property on="ok" class="Bool"("Visible"=w1) -> ()  [unwired: 2 in, 2 out]
      n4 = Build Array("peak #", "time (min)", "peak area") -> (w5:string[])
      n5 = property on="table" class="Tbl (strict)"("Column Header Strings[]"=w5) -> ()  [unwired: 2 in, 2 out]
    }
    frame #1 {
      n6 = while {
        stop <- w15 continue-if-true
        n7 = Transpose 2D Array(2D array="table in") -> (transposed array=w11:string[][])
        n8 = Array Size(array=w11) -> (size(s)=w9:i32[])
        n9 = Index Array(array=w9, index=0) -> (element=w8:i32)
        n10 = Array Subset(array=w11, index (row)=0, length (row)=w8, index (col)=1, length (col)=3) -> (→"table":string[][])
        n11 = Not(x="ok") -> (.not. x?=w15:bool)
      }
    }
    frame #2 {
      w17 = FALSE
      n12 = property on="ok" class="Bool"("Visible"=w17) -> ()  [unwired: 2 in, 2 out]
      n13 = property on="peaks graph 1" class="XYGraph (strict)"("Palette:Visible"=w17) -> ()  [unwired: 2 in, 2 out]
    }
  }
